vi "TLB Native Dynamic Events ver 0.15b.vi"() -> ()   [LabVIEW 2018]
uses:
  Labview Training Phase 2/Enum Controls/States for Action Engine.ctl
  TLB Type Definitions/State Type Definitions.ctl
  TLB Type Definitions/Intruction Type Definitions.ctl
  TLB Type Definitions/Encoder cluster.ctl
  TLB Type Definitions/PING CLUSTER.ctl
  <vilib>/Studica/Studica Toolkit/NavX/NavX.lvlib
  <vilib>/Studica/Studica Toolkit/Background/DIO Channel.ctl
  Underlying VI's/NavX VI/navX type def.ctl
  <vilib>/myRIO/Instrument Drivers/Utilities/Utilities.lvlib
  <vilib>/Studica/Studica Toolkit/Background/I2C Channel.ctl
  TLB Type Definitions/Vision cluster.ctl
  <vilib>/NI_Real-Time Target Support.lvlib
  TLB Type Definitions/Stepper cluster.ctl
  Experimental VI's/Archived VI's/MOTOR CONTROL NO PID Type Def.ctl
  Underlying VI's/I2C Master VI/I2C MASTER Type Def.ctl
  Underlying VI's/I2C Master VI/I2C_MASTER_WRITE_NEW Type Def.ctl
  <vilib>/userdefined/High Color/IMAQdx.ctl
  Underlying VI's/I2C Master VI/Arduino_Interfacing.ctl
  TLB Type Definitions/Yaw Cluster.ctl
  Experimental VI's/Archived VI's/MOTOR CONTROL NO PID AE DATA ENTRY MODE Type def.ctl
  Experimental VI's/Archived VI's/MOTOR CONTROL NO PID AE DIRECTIONS type def.ctl
  TLB Type Definitions/Time cluster.ctl
  TLB Type Definitions/Y Stepper cluster.ctl
  Underlying VI's/Modified webcam FGV/Webcam AE.ctl
  Underlying VI's/Elasped Timer/Elapsed timer control.ctl
  <vilib>/Utility/RT CPU Load.ctl
panel:
  out "Object Center Coordinates":cluster{"x":sgl, "y":sgl}
  out "Object detection cluster":T1
  out "Time up flag":bool
  out "Speed & distance":T2
  out "Task selection":u8
  in  "Object recognition mode":enum16{"Ball", "Soap", "Gel", "Pipe", "None"}(ring)
  out "NavX Readings":T3
  out "Arduino Data":T4
  out "CPU loads":T5[](array[typedef]) {"ISR (%)" format="%#.2f"; "Idle (%)" format="%#.2f"; "Background (%)" format="%#.2f"; "Normal (%)" format="%#.2f"; "Above Normal (%)" format="%#.2f"; "High (%)" format="%#.2g"; "Timed Structures (%)" format="%#.2g"; "Time Critical (%)" format="%#.2g"; "Total (%)" format="%#.2g"}
  out "TASK ENABLE":bool
  out "Rising Edge":bool
  in  "Green LED":bool
  out "Obstacle detected":bool
  out "I2C Error":errorcluster
  out "State Logic":T6=enum."Startup"
  out "elements":T7[](array[typedef])
  in  "STOP TASK":bool
  in  "OK Button":bool
  in  "STOP":bool
  out "error out":errorcluster
  out "Action Queue Items":i32
  out "State Logic Queue Items":i32
  out "Action Queues items":string[](array[string])=["Hardware reset", "Software reset", ""]
  out "Action State":string
  # "System Health Status Update"
  # "VISION"
  # "TLB FRAMEWORK STATUS"
  # "Test Programme written by Calvin Loke    Dated: 28 Aug 2019\nTest Programme revised by Dr Alex See   Dated 30 Aug 2019\n\nRevision date: 20/03/2020\nProgramme version:   TLB Native Dynamic Events ver 0.14a"
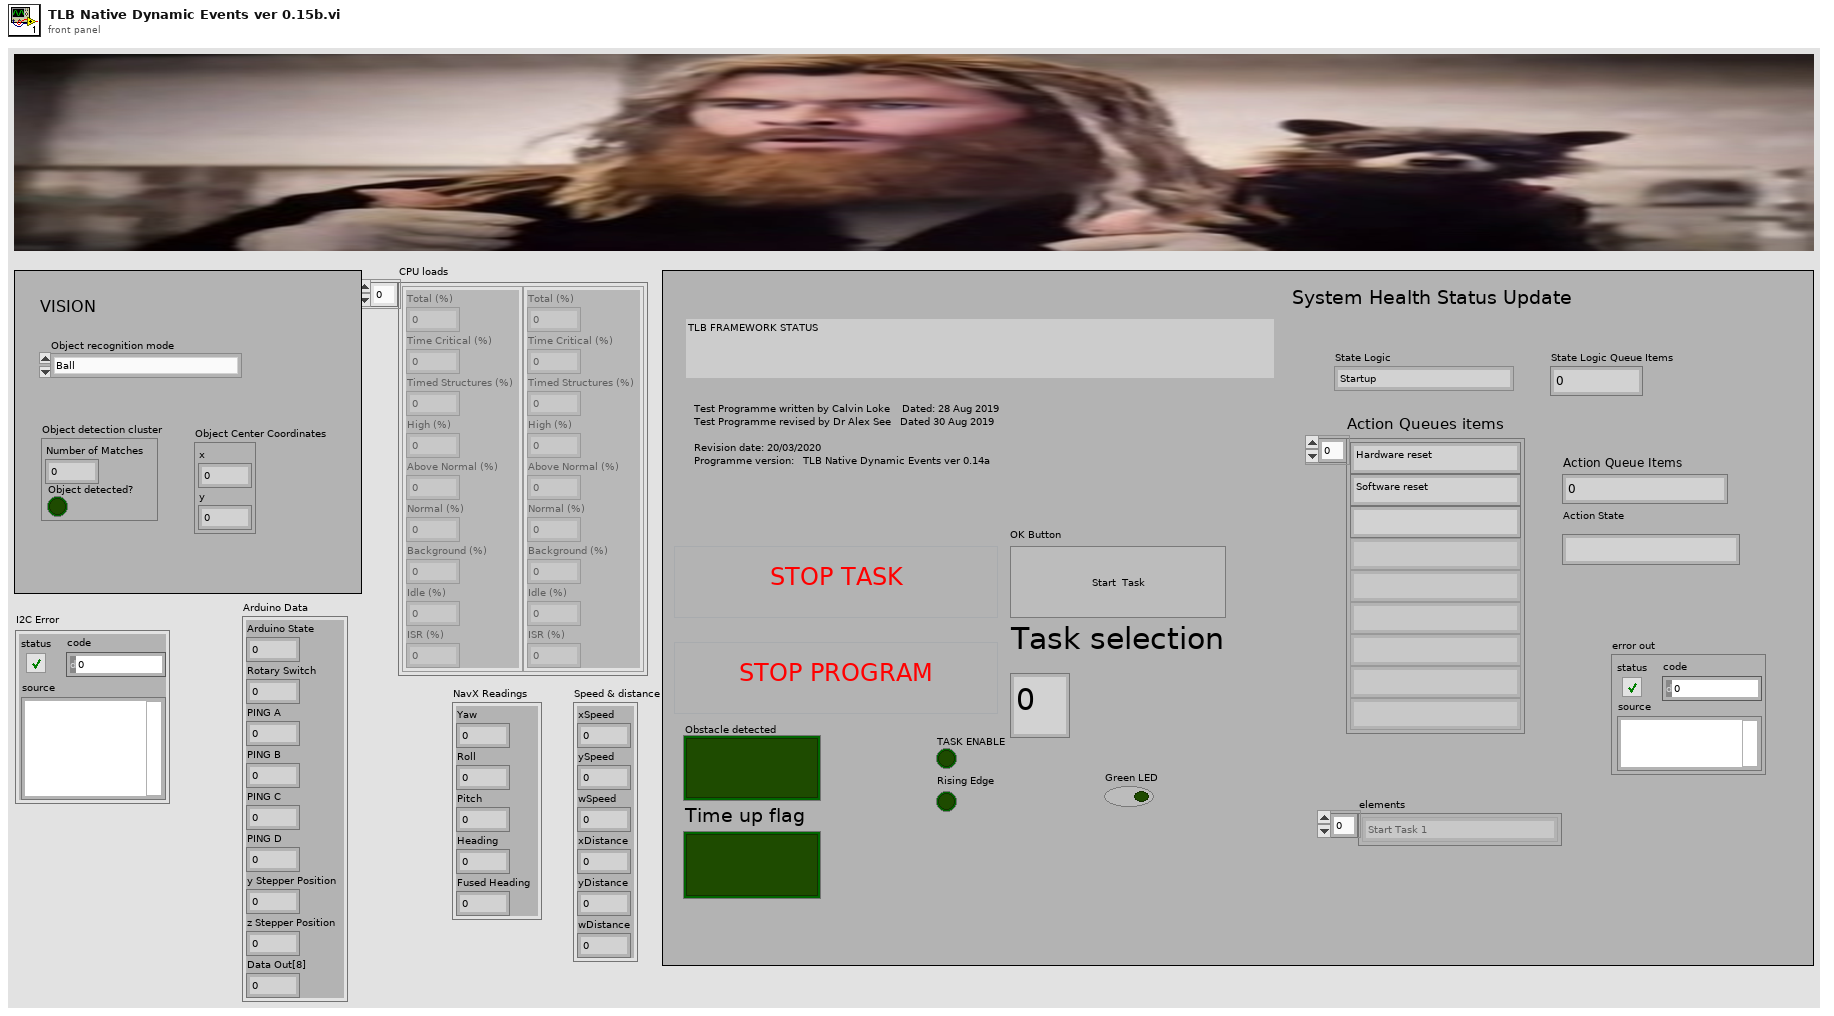
[diagram p1: front panel]
types:
  T1 = cluster{"Number of Matches":i32, "Object detected?":bool}
  T2 = cluster{"xSpeed":dbl, "ySpeed":dbl, "wSpeed":dbl, "xDistance":dbl, "yDistance":dbl, "wDistance":dbl}
  T3 = cluster{"Yaw":dbl, "Roll":dbl, "Pitch":dbl, "Heading":dbl, "Fused Heading":dbl}
  T4 = cluster{"Arduino State":u8, "Rotary Switch":u8, "PING A":u8, "PING B":u8, "PING C":u8, "PING D":u8, "y Stepper Position":u8, "z Stepper Position":u8, "Data Out[8]":u8}
  T5 = typedef "NI_Real-Time Target Support.lvlib/RT CPU Load.ctl" = cluster{"Total (%)":dbl, "Time Critical (%)":dbl, "Timed Structures (%)":dbl, "High (%)":dbl, "Above Normal (%)":dbl, "Normal (%)":dbl, "Background (%)":dbl, "Idle (%)":dbl, "ISR (%)":dbl}
  T6 = typedef "State Type Definitions.ctl" = enum16{"None", "Startup", "Move to Angle", "True Stop", "Idle", "Shutdown", "Task 1A", "Task 1B", "Task 2:Raise Arm", "Task 2:Sensor Mode", "Task 2:Reverse Mode", "Task 3", "Task 4_A", "Task 4_B", "Task 4_C", "Task 4_D", "Task 5A", "Task 5B", "Task 5C", "Task 5D", "Task 5E: POSITION ARM", "Task 5F: ARM GRAB HEIGHT", "Task 5G: CLOSE CLAW", "Task 5H: RAISE ARM", "Task 6_A", "Task 6_B", "Task 7", "Task 8A: RAISE ARM", "Task 8B: MOVE TO BOX", "Task 8C: CAM BURST", "Task 8D: PROCESS IMAGE", "Task 8E: ROBOT ADJUST", "Task 8F: CAM BURST 2", "Task 8G: PROCESS IMAGE 2", "Task 8H: ARM ADJUST", "Task 8I: ARM GRAB HEIGHT", "Task 8J: CLOSE CLAW", "Task 8K: RAISE MY SWORD", "Task 9A: Raise Arm", "Task 9B: Rotate to Angle", "Task 9C: Detect Box", "Task 9D: MOVE FORWARD", "Task 9E: MOVE LEFT", "Task 9F: SCAN IMAGE", "Task 9G: PROCESS COLOUR", "Task 9H: MOVE RIGHT", "Task 9I: SCAN IMAGE", "Task 9J: PROCESS COLOUR", "Task 9K: ROTATE 90 CW", "Task 9L: MOVE FORWARD", "Task 9M: MOVE RIGHT", "Task 9N: SCAN IMAGE", "Task 9O: PROCESS COLOUR", "Task 9P: MOVE RIGHT", "Task 9Q: SCAN IMAGE", "Task 9R: PROCESS COLOUR", "Task A1: Raise Arm", "Task A2: Rotate to Angle", "Task A3: Move Forward", "Task A4: Rotate CW 90"}
  T7 = typedef "Intruction Type Definitions.ctl" = enum16{"None", "Start Task 1", "Start Task 2", "Start Task 3", "Start Task 4", "Start Task 5", "Start Task 6", "Start Task 7", "Start Task 8 - BALL", "Start Task 8 - Gel", "Start Task 8 - Pipe", "Start Task 8 - Soap", "Start Task 9", "Start Task A", "Start Task B", "Exit"}
  T8 = typedef "Y Stepper cluster.ctl" = cluster{"yStepper desired":u8}
  T9 = typedef "Time cluster.ctl" = cluster{"Time up flag":bool, "SET TIME TO CHECK":dbl}
  T10 = typedef "Yaw Cluster.ctl" = cluster{"Yaw":dbl, "Compass":dbl}
  T11 = typedef "Stepper cluster.ctl" = cluster{"y Stepper Position":u8, "z Stepper Position":u8}
  T12 = typedef "DIO Channel.ctl" = enum16{"Not Connected", "A/DIO1", "A/DIO2", "A/DIO3", "A/DIO4", "A/DIO5", "A/DIO6", "A/DIO7", "A/DIO13", "B/DIO1", "B/DIO2", "B/DIO3", "B/DIO4", "B/DIO5", "B/DIO6", "B/DIO7", "B/DIO13", "C/DIO0", "C/DIO1", "C/DIO2", "C/DIO3", "C/DIO4", "C/DIO5", "C/DIO6", "C/DIO7"}
  T13 = typedef "Vision cluster.ctl" = cluster{"Recognized Object":bool, "Object X coordinate":dbl, "Object Y coordinate":dbl}
  T14 = typedef "PING CLUSTER.ctl" = cluster{"PING_A":u8, "PING_B":u8, "PING_C":u8, "PING_D":u8}
  T15 = typedef "Encoder cluster.ctl" = cluster{"xDistance":dbl, "yDistance":dbl, "wDistance":dbl}
  T16 = cluster{"DIO Channel":T12, "FPGA VI Reference Out":refnum<k20>}
  T17 = typedef "MOTOR CONTROL NO PID AE DATA ENTRY MODE Type def.ctl" = enum16{"Initialize", "Reset Encoders", "Write to motors", "Read from Encoders"}
  T18 = typedef "navX type def.ctl" = enum16{"Get i2C reference", "Read Values", "Zero Yaw"}
  T19 = typedef "Arduino_Interfacing.ctl" = enum16{"Initialize", "Write to Arduino", "Read From Arduino"}
  T20 = typedef "I2C Channel.ctl" = enum16{"Not Connected", "A", "B"}
  T21 = typedef "States for Action Engine.ctl" = enum16{"Initialize", "Write", "Read"}
  T22 = cluster{"I2C Ref Out":cluster{"I2C Channel":T20, "FPGA VI Reference Out":refnum<k20>}, "Connected":bool, "Slave Address (7-bit)":u8, "Registry":u8[]}
  T23 = typedef "IMAQ Image.ctl" = refnum<image>
  T24 = typedef "State Type Definitions.ctl" = enum16{"None", "Startup", "Move to Angle", "True Stop", "Idle", "Shutdown", "Task 1", "Task 2", "Task 3", "Task 4_A", "Task 4_B", "Task 4_C", "Task 4_D", "Task 5_A", "Task 5 _B", "Task 5_C", "Task 5_D", "Task 5_D_Error", "Task 5D_Error_Right", "Task 5D_Error_Left", "Task 5_E", "Task 5_F", "Task 5F_Error", "Task 5G", "Task 5H", "Task 5I", "Task 6_A", "Task 6_B", "Task 7", "Task 8", "Task 9", "Task A", "Task B"}
  T25 = typedef "MOTOR CONTROL NO PID AE DIRECTIONS type def.ctl" = enum16{"y-axis movement", "x-axis movement", "Rotate", "Stop"}
  T26 = typedef "Elapsed timer control.ctl" = enum16{"Start", "Pause", "Initialize"}
  T27 = typedef "I2C_MASTER_WRITE_NEW Type Def.ctl" = enum16{"Ultrasonic sensors", "Stepper origin", "zStepper 13.3k", "zStepper 13k", "zStepper 12k", "zStepper 11k", "zStepper 10k", "zStepper 9k", "zStepper 8k", "zStepper 7k", "zStepper 6k", "zStepper 5k", "zStepper 4k", "zStepper 3k", "zStepper 2k", "zStepper 1k", "zStepper 900", "zStepper 800", "zStepper 700", "zStepper 600", "zStepper 500", "zStepper 400", "zStepper 300", "zStepper 200", "zStepper 100", "zStepper 0", "yStepper control", "Open Claw", "Close Claw", "Soft Reset"}
  T28 = typedef "Webcam AE.ctl" = enum16{"Initialize Camera", "Open Camera", "Continuous Acquisition", "Close Camera", "Retrieve Image", "Dispose Camera Image Buffer"}
  T29 = typedef "IMAQdx.ctl" = refnum<k21>
  T30 = typedef "Webcam AE.ctl" = enum16{"Initialize Camera", "Open Camera", "Continuous Acquisition", "Close Camera", "Retrieve Image", "Dispose Image Buffers"}
  T31 = typedef "MOTOR CONTROL NO PID Type Def.ctl" = enum16{"Init", "Front Back", "Left Right", "Rotate", "Stop", "Latch"}
  T32 = typedef "I2C MASTER Type Def.ctl" = enum16{"Last State", "Mode 0", "Mode 1", "Mode 2", "Mode 3", "Mode 4", "Mode 5", "Mode 6", "Mode 7", "Mode 8", "Mode 9", "Mode 10"}
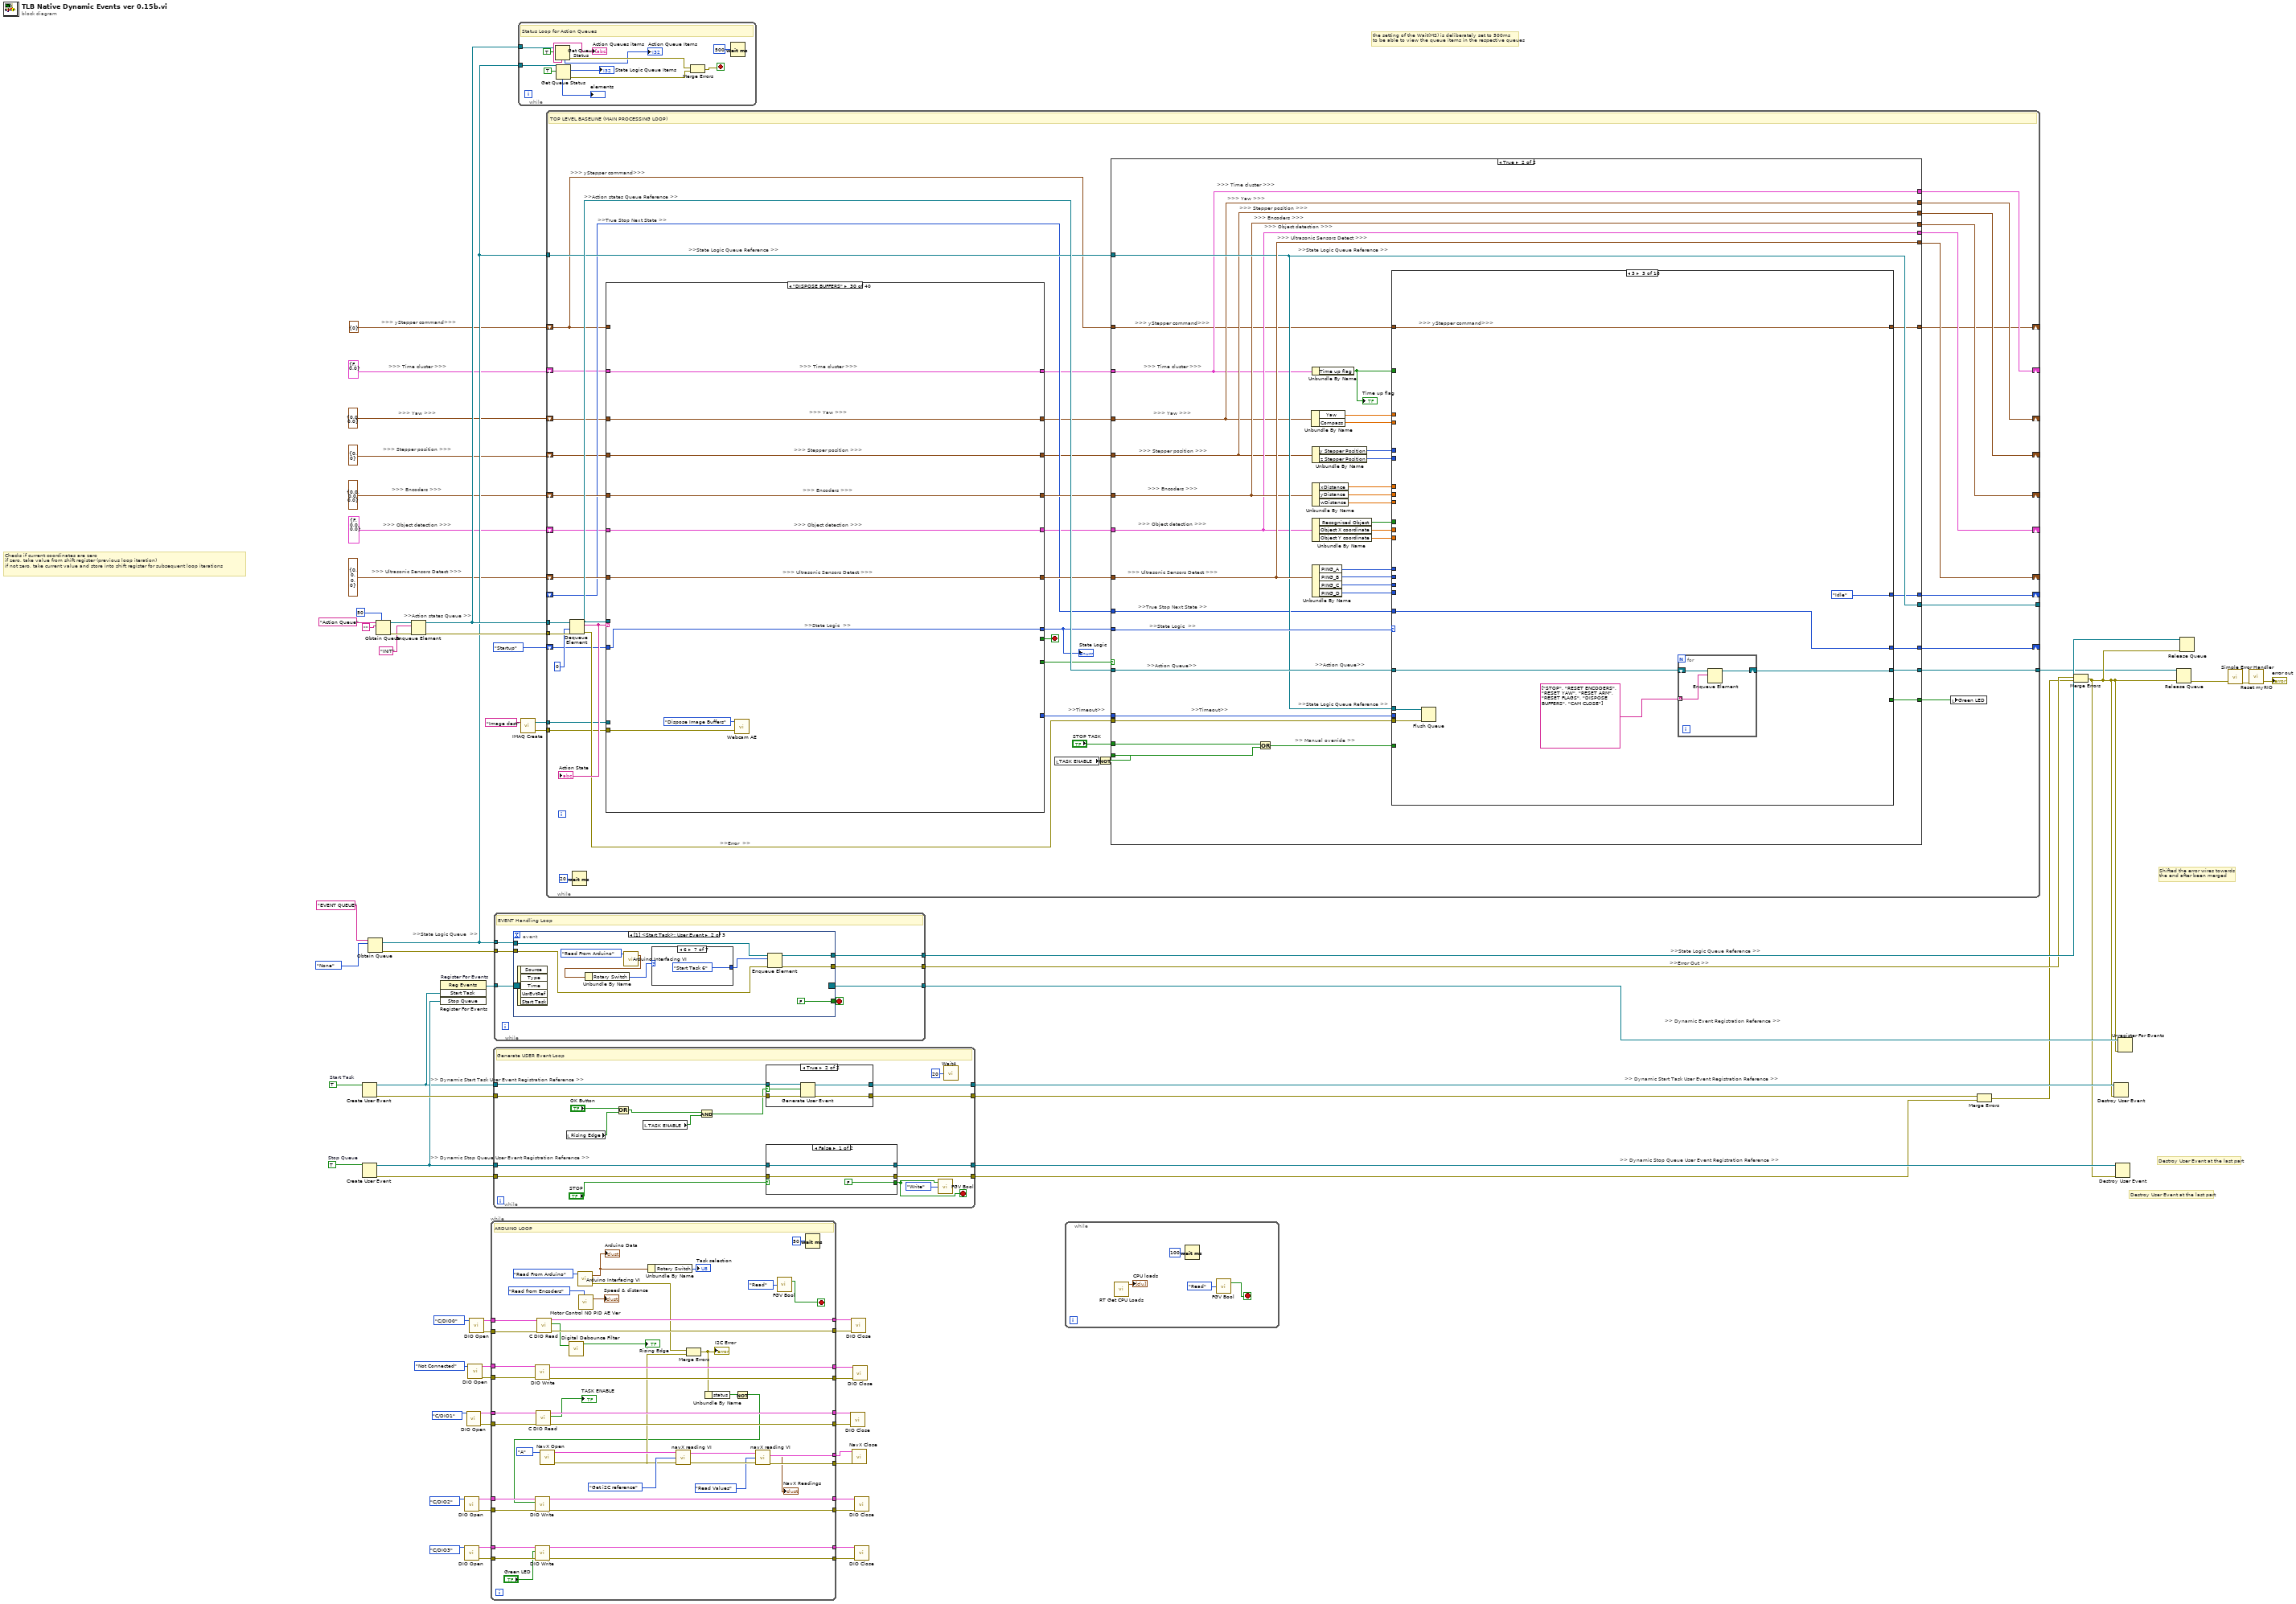
[diagram p0: block diagram]
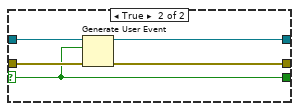
[diagram p2: hidden frame]
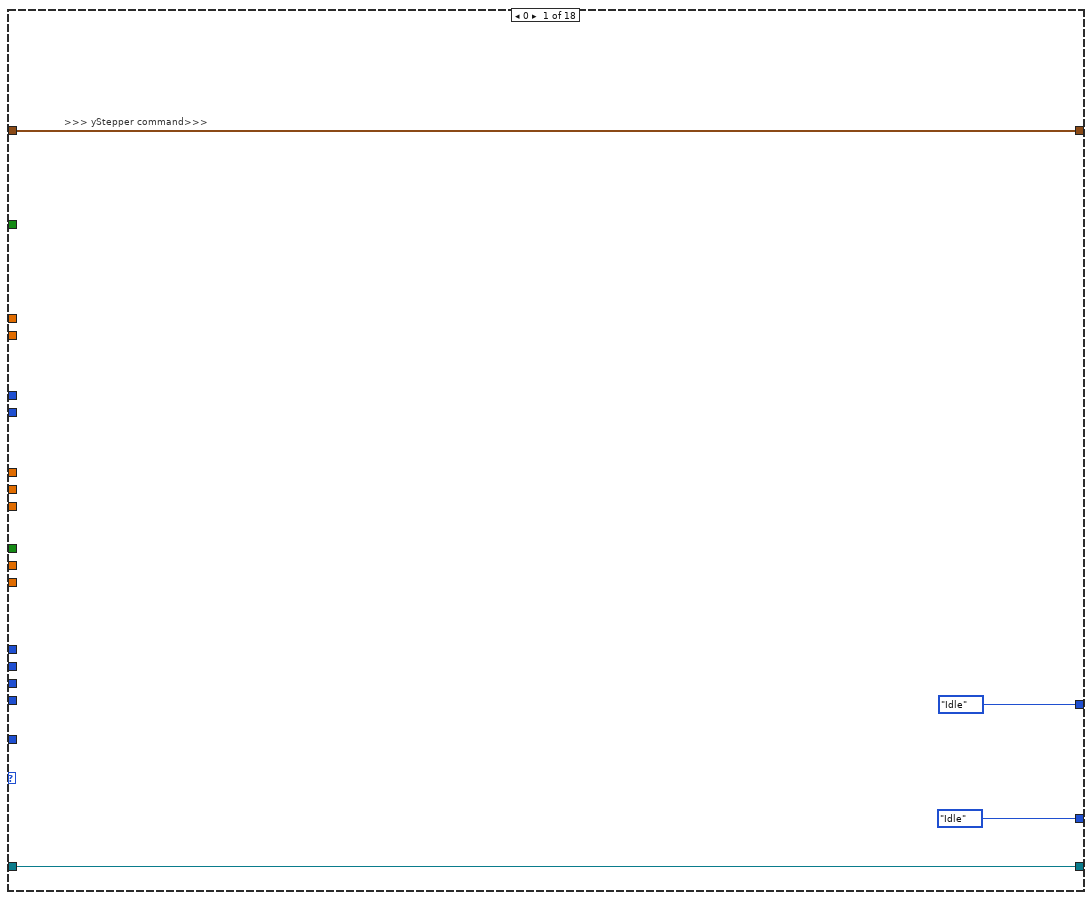
[diagram p5: hidden frame]
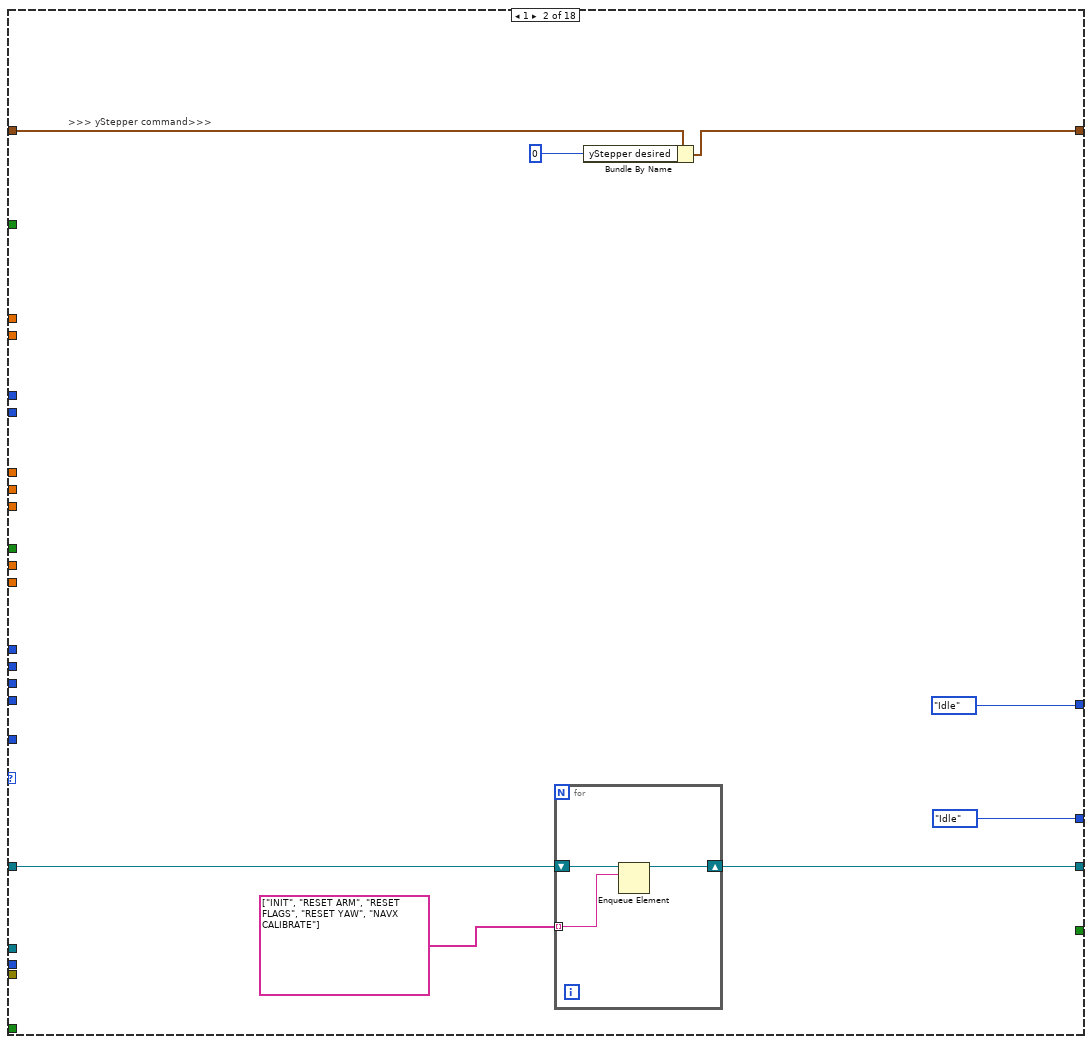
[diagram p6: hidden frame]
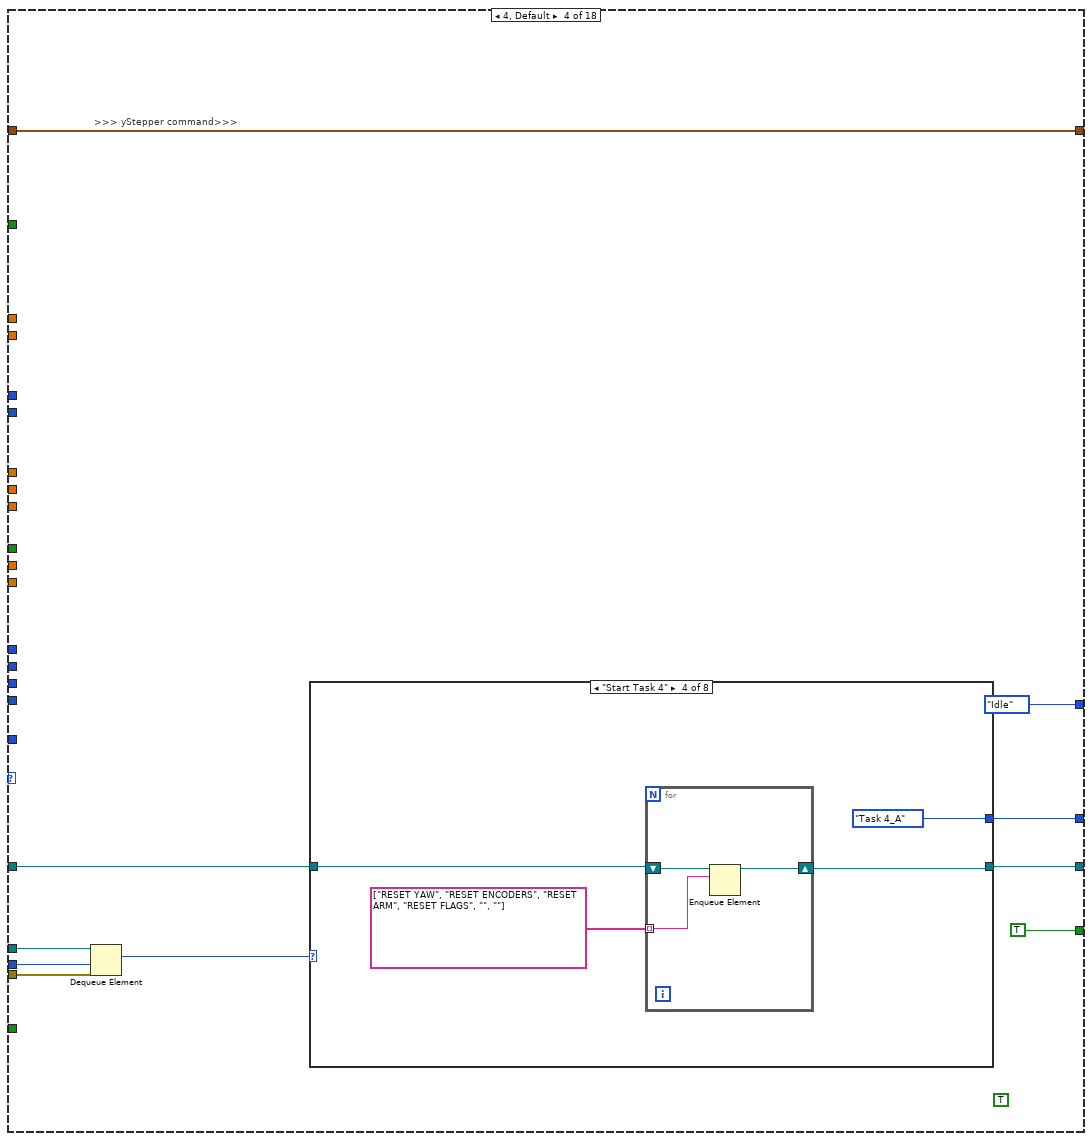
[diagram p7: hidden frame]
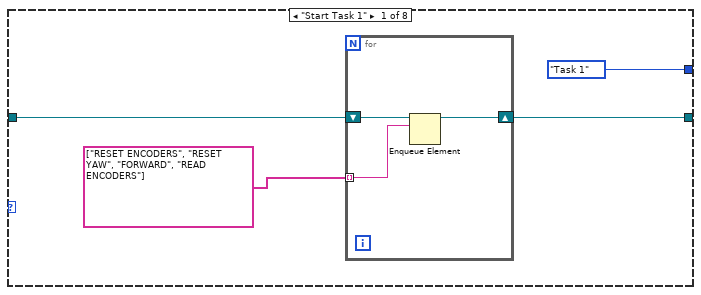
[diagram p8: hidden frame]
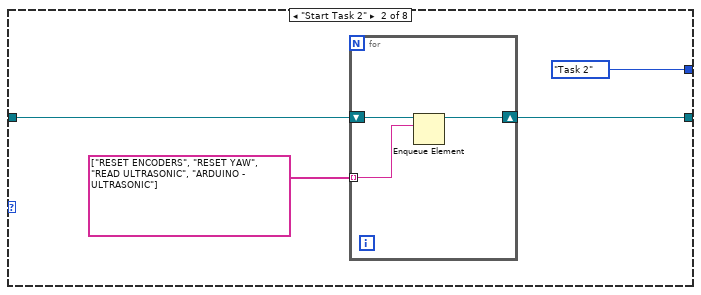
[diagram p9: hidden frame]
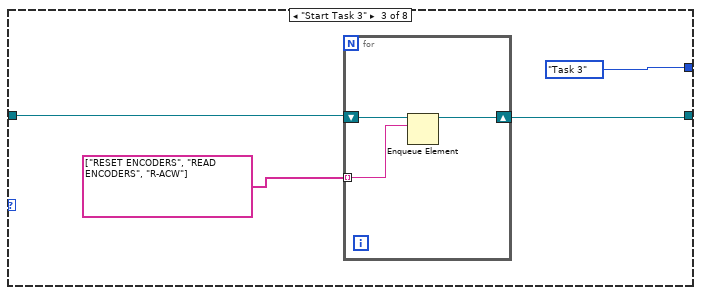
[diagram p10: hidden frame]
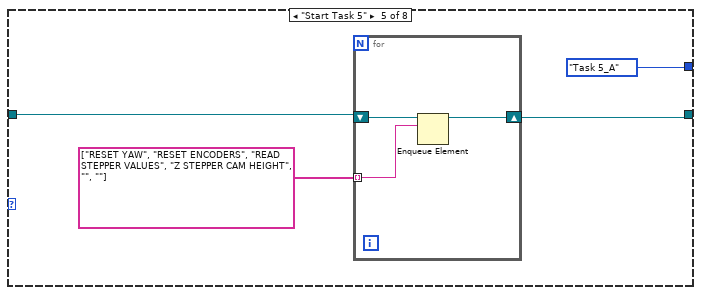
[diagram p11: hidden frame]
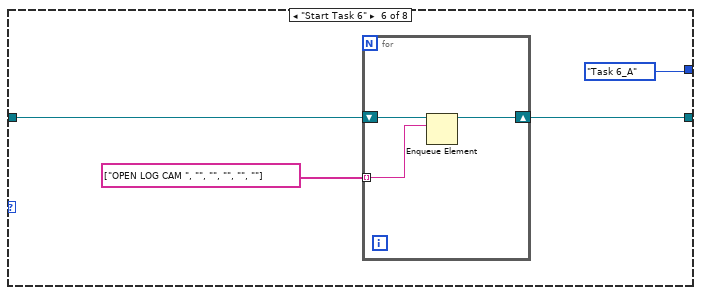
[diagram p12: hidden frame]
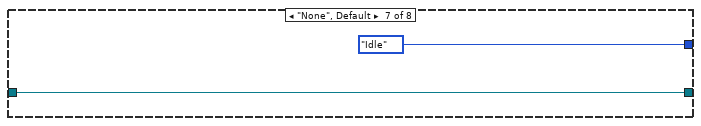
[diagram p13: hidden frame]
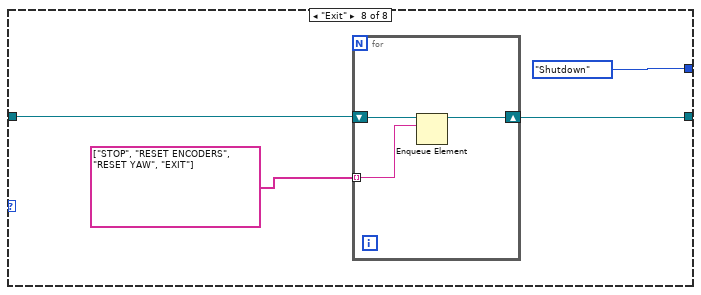
[diagram p14: hidden frame]
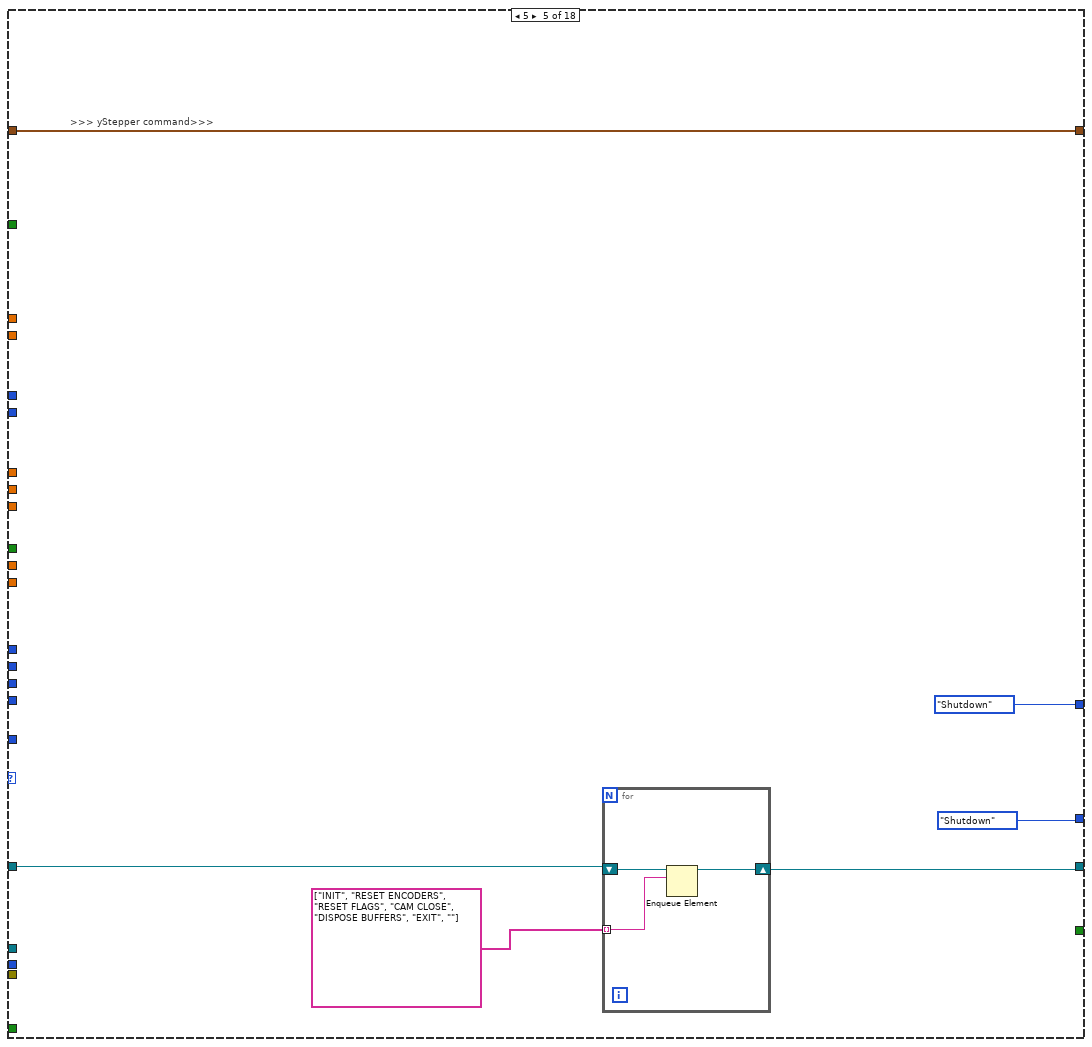
[diagram p15: hidden frame]
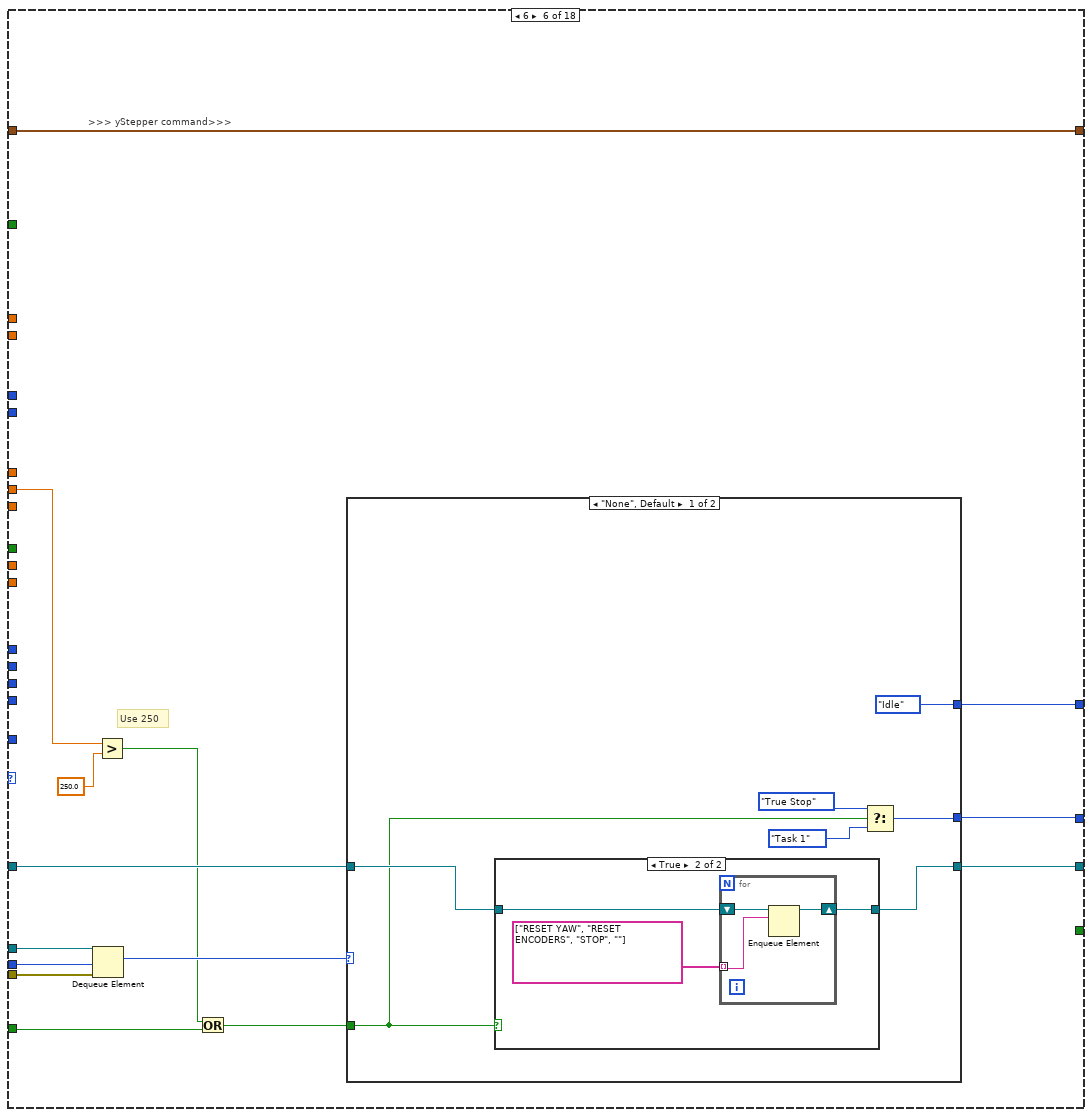
[diagram p16: hidden frame]
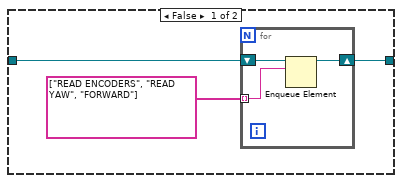
[diagram p17: hidden frame]
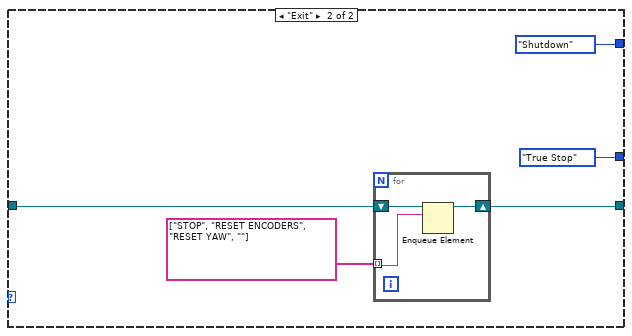
[diagram p18: hidden frame]
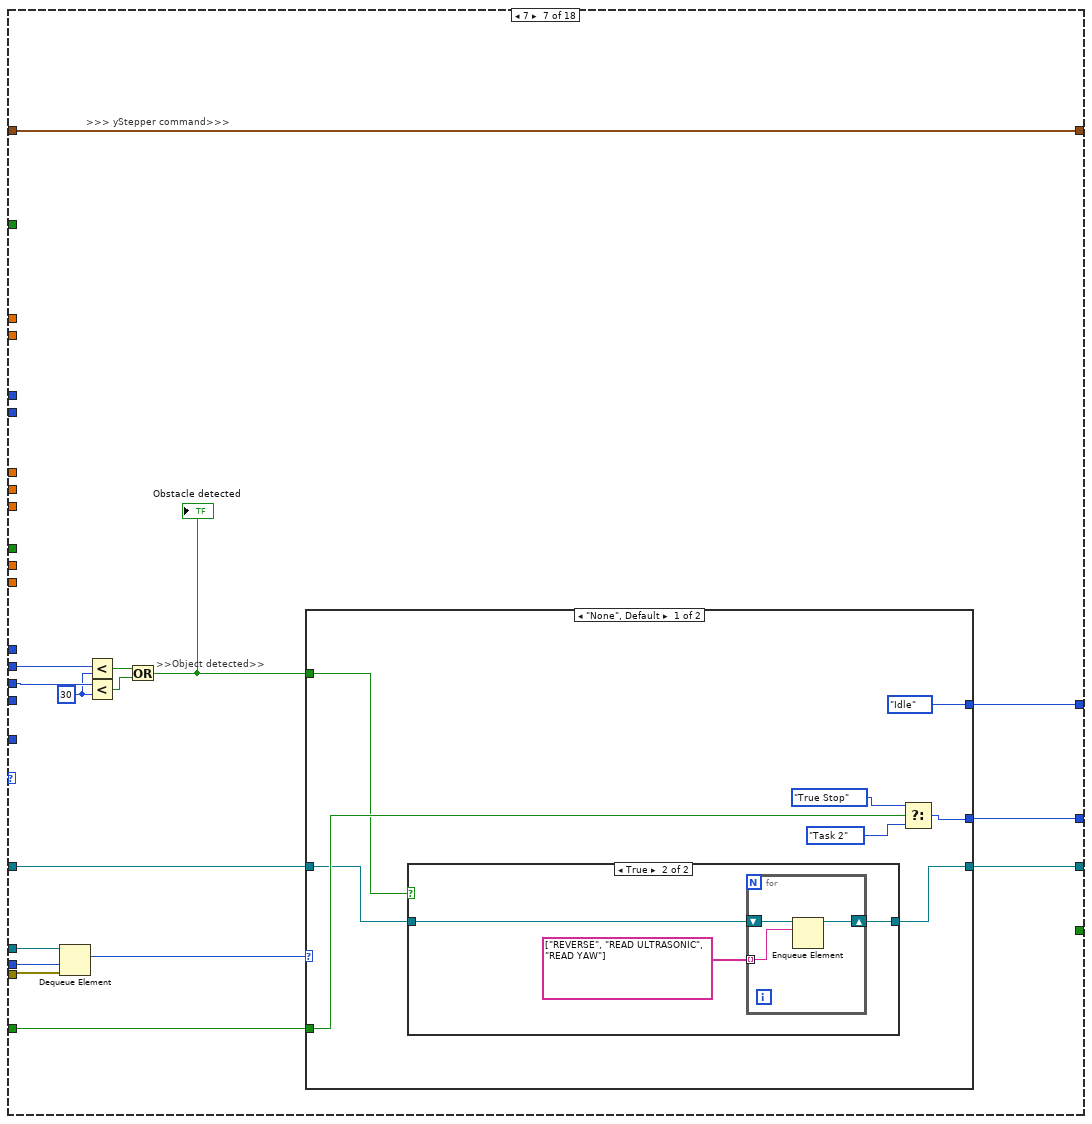
[diagram p19: hidden frame]
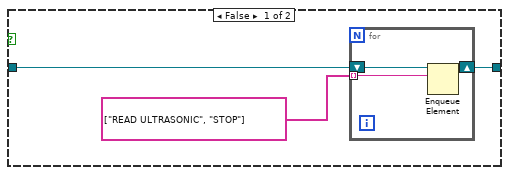
[diagram p20: hidden frame]
diagram:
  w70 = TRUE  # Stop Queue
  w69 = TRUE  # Start Task
  # "Checks if current coordinates are zero\nif zero, take value from shift register (previous loop iteration)\nif not zero, take current value and store into shift register for subsequent loop iterations"
  # ">>> yStepper command>>>"
  # ">>> Time cluster >>>"
  # ">>> Yaw >>>"
  # ">>> Stepper position >>>"
  # ">>> Encoders >>>"
  # ">>> Object detection >>>"
  # ">>> Ultrasonic Sensors Detect >>>"
  # "the setting of the Wait(MS) is deliberately set to 500ms\nto be able to view the queue items in the respective queues"
  # ">>Error Out >>"
  # ">> Dynamic Stop Queue User Event Registration Reference >>"
  # ">> Dynamic Start Task User Event Registration Reference >>"
  # ">> Dynamic Stop Queue User Event Registration Reference >>"
  # ">> Dynamic Start Task User Event Registration Reference >>"
  # ">> Dynamic Event Registration Reference >>"
  # ">>Action states Queue >>"
  # ">>State Logic Queue  >>"
  # ">>State Logic Queue Reference >>"
  # "Destroy User Event at the last part"
  # "Destroy User Event at the last part"
  # "Shifted the error wires towards\nthe end after been merged"
  n1 = Create User Event(user event datatype=w69) -> (user event=w61:refnum<user-event>, error out=w66:errorcluster)  [unwired: 1 in]
  n2 = Create User Event(user event datatype=w70) -> (user event=w62:refnum<user-event>, error out=w65:errorcluster)  [unwired: 1 in]
  n3 = Obtain Queue(name (unnamed)="EVENT QUEUE", element data type=Intruction_Type_Definitions."None" ("Enum")) -> (queue out=w47:refnum<queue>, error out=w53:errorcluster)  [unwired: 3 in, 1 out]
  n4 = Obtain Queue(max queue size (-1, unlimited)=50, name (unnamed)="Action Queue", element data type="") -> (queue out=w56:refnum<queue>, error out=w52:errorcluster)  [unwired: 2 in, 1 out]
  n5 = Enqueue Element(queue=w56, element="INIT", error in (no error)=w52) -> (queue out=w48:refnum<queue>, error out=w51:errorcluster)  [unwired: 1 in, 1 out]
  n6 = register-events "Register For Events"(w61, w62) -> (reference out=w60:refnum<event-registration>)  [unwired: 2 in, 1 out]
  n7 = call <vilib>:"DIO Open.vi"("DIO Channel"=DIO_Channel."C/DIO2") -> ("error out"=w14:errorcluster, "DIO Info Out"=w15:T16)  [unwired: 9 in]
  n8 = call <vilib>:"DIO Open.vi"("DIO Channel"=DIO_Channel."C/DIO3") -> ("error out"=w9:errorcluster, "DIO Info Out"=w10:T16)  [unwired: 9 in]
  n9 = call <vilib>:"DIO Open.vi"("DIO Channel"=DIO_Channel."C/DIO1") -> ("error out"=w25:errorcluster, "DIO Info Out"=w26:T16)  [unwired: 9 in]
  n10 = call <vilib>:"DIO Open.vi"("DIO Channel"=DIO_Channel."Not Connected") -> ("error out"=w30:errorcluster, "DIO Info Out"=w32:T16)  [unwired: 9 in]
  n11 = call <vilib>:"DIO Open.vi"("DIO Channel"=DIO_Channel."C/DIO0") -> ("error out"=w35:errorcluster, "DIO Info Out"=w38:T16)  [unwired: 9 in]
  n12 = while {
    tunnel: w38 -> [w113]
    tunnel: [w112] -> w36
    tunnel: w35 -> [w111]
    tunnel: [w110] -> w34
    tunnel: w32 -> [w107]
    tunnel: [w106] -> w31
    tunnel: w30 -> [w105]
    tunnel: [w104] -> w29
    tunnel: [w103] -> w27
    tunnel: w26 -> [w102]
    tunnel: w25 -> [w101]
    tunnel: [w100] -> w24
    tunnel: w15 -> [w94]
    tunnel: w14 -> [w93]
    tunnel: [w92] -> w13
    tunnel: [w91] -> w12
    tunnel: w10 -> [w90]
    tunnel: w9 -> [w89]
    tunnel: [w88] -> w8
    tunnel: [w87] -> w7
    tunnel: [w81] -> w4
    tunnel: [w80] -> w5
    stop <- w115 stop-if-true
    # "ARDUINO LOOP"
    n13 = call <vilib>:"DIO Write.vi"("error in (no error)"=w89, "Input"="Green LED", "DIO Info In"=w90) -> ("error out"=w87:errorcluster, "DIO Info Out"=w88:T16)  [unwired: 7 in]
    n14 = call <vilib>:"DIO Write.vi"("error in (no error)"=w105, "DIO Info In"=w107) -> ("error out"=w104:errorcluster, "DIO Info Out"=w106:T16)  [unwired: 8 in]
    n15 = call <vilib>:"C DIO Read.vi"("error in (no error)"=w101, "DIO Info In in"=w102) -> ("error out"=w100:errorcluster, "IN"=→"TASK ENABLE":bool, "DIO Info In out"=w103:T16)  [unwired: 7 in]
    n16 = call <vilib>:"C DIO Read.vi"("error in (no error)"=w111, "DIO Info In in"=w113) -> ("error out"=w110:errorcluster, "IN"=w109:bool, "DIO Info In out"=w112:T16)  [unwired: 7 in]
    n17 = call <vilib>:"NavX Open.vi"("I2C Channel"=I2C_Channel."A") -> ("error out"=w96:errorcluster, "NavX Info"=w98:T22)  [unwired: 9 in]
    n18 = call "Digital Debounce Filter.vi"("Boolean input"=w109) -> ("Rising Edge"=→"Rising Edge":bool)  [unwired: 1 in, 2 out]
    n19 = call "Arduino Interfacing VI.vi"("AE Mode"=Arduino_Interfacing."Read From Arduino") -> ("error out"=w84:errorcluster, "Arduino Data"=w77:T4)  [unwired: 3 in]
    "Arduino Data" <- w77
    n20 = call "Motor Control NO PID AE Ver.vi"("AE Mode"=MOTOR_CONTROL_NO_PID_AE_DATA_ENTRY_MODE_Type_def."Read from Encoders") -> ("Speed & distance"=→"Speed & distance":T2)  [unwired: 4 in, 1 out]
    n21 = Unbundle By Name(w77) -> ("Rotary Switch"=→"Task selection":u8)
    n22 = call "navX reading VI.vi"("NavX Info In"=w98, "Mode"=navX_type_def."Get i2C reference", "error in (no error)"=w96) -> ("NavX Info Out"=w83:T22, "Error Out"=w82:errorcluster)  [unwired: 2 out]
    n23 = Merge Errors(w84, w96) -> (w73:errorcluster)
    "I2C Error" <- w73
    n24 = Unbundle By Name(w73) -> ("status"=w72:bool)
    n25 = Not(x=w72) -> (.not. x?=w71:bool)
    n26 = call <vilib>:"DIO Write.vi"("error in (no error)"=w93, "Input"=w71, "DIO Info In"=w94) -> ("error out"=w91:errorcluster, "DIO Info Out"=w92:T16)  [unwired: 7 in]
    n27 = call "navX reading VI.vi"("NavX Info In"=w83, "Mode"=navX_type_def."Read Values", "error in (no error)"=w82) -> ("NavX Info Out"=w81:T22, "NavX Readings"=→"NavX Readings":T3, "Error Out"=w80:errorcluster)  [unwired: 1 out]
    n28 = call "FGV Bool.vi"("Init/Read/Write State"=States_for_Action_Engine."Read") -> ("Output node"=w115:bool)  [unwired: 2 in, 1 out]
    n29 = Wait (ms)(milliseconds to wait=u32 50) -> ()  [unwired: 1 out]
  }
  n30 = while {
    tunnel: w61 -> [w133]
    tunnel: w62 -> [w132]
    tunnel: [w131] -> w68
    tunnel: [w130] -> w67
    tunnel: w66 -> [w129]
    tunnel: [w128] -> w64
    tunnel: w65 -> [w127]
    tunnel: [w126] -> w63
    stop <- w124 stop-if-true
    # "Generate USER Event Loop"
    n31 = local read "Rising Edge"() -> (w120:bool)
    n32 = Or(x="OK Button", y=w120) -> (x .or. y?=w119:bool)
    n33 = local read "TASK ENABLE"() -> (w118:bool)
    n34 = And(x=w119, y=w118) -> (x .and. y?=w117:bool)
    n35 = case shown="True" w117 {
      selector: w117 -> [_ w144]
      tunnel: w133 -> [w143 w148]
      tunnel: [w143 w147] -> w130
      tunnel: w129 -> [w142 w146]
      tunnel: [w142 w145] -> w128
      frame False {
      }
      frame True {
        n36 = Generate User Event(user event=w148, event data cluster=w144, error in=w146) -> (user event out=w147:refnum<user-event>, error out=w145:errorcluster)  [unwired: 1 in]
      }
    }
    n37 = case shown="False" "STOP" {
      selector: "STOP" -> [_ w137]
      tunnel: w132 -> [w136 w141]
      tunnel: [w136 w140] -> w131
      tunnel: w127 -> [w135 w139]
      tunnel: [w135 w138] -> w126
      tunnel: [FALSE w137] -> w124
      frame False {
      }
      frame True {
        n38 = Generate User Event(user event=w141, event data cluster=w137, error in=w139) -> (user event out=w140:refnum<user-event>, error out=w138:errorcluster)  [unwired: 1 in]
      }
    }
    n39 = call "FGV Bool.vi"("Init/Read/Write State"=States_for_Action_Engine."Write", "Input Node"=w124) -> ()  [unwired: 1 in, 2 out]
    n40 = call "Wait4"("Count(uSec)"=u32 20) -> ()  [unwired: 1 out]
  }
  n41 = while {
    tunnel: w60 -> [w155]
    tunnel: [w154] -> w59
    tunnel: w47 -> [w152]
    tunnel: [w151] -> w58
    tunnel: w53 -> [w150]
    tunnel: [w149] -> w50
    stop <- w153 stop-if-true
    # "EVENT Handling Loop"
    n42 = event shown="[1] <Start Task>: User Event" {
      selector: w155 -> [_ _ _]
      dyn-events: [_ _ _] -> w154
      timeout: _ -> [_ _ _]
      tunnel: [FALSE FALSE w183] -> w153
      tunnel: w152 -> [w160 w169 w181]
      tunnel: [w159 w168 w182] -> w151
      tunnel: w150 -> [w158 w167 w180]
      tunnel: [w157 w166 w179] -> w149
      event Timeout {
        n43 = event-data() -> ()  [unwired: 1 in, 3 out]
        n44 = Enqueue Element(queue=w160, element=Intruction_Type_Definitions."None" ("Enum"), error in (no error)=w158) -> (queue out=w159:refnum<queue>, error out=w157:errorcluster)  [unwired: 1 in, 1 out]
      }
      event User Event {
        n45 = event-data() -> ()  [unwired: 1 in, 5 out]
        n46 = call "Arduino Interfacing VI.vi"("AE Mode"=Arduino_Interfacing."Read From Arduino") -> ("Arduino Data"=w163:T4)  [unwired: 3 in, 1 out]
        n47 = Unbundle By Name(w163) -> ("Rotary Switch"=w162:u8)
        n48 = case shown="6" w162 {
          tunnel: [Intruction_Type_Definitions."None" ("Enum") Intruction_Type_Definitions."Start Task 1" ("Enum") Intruction_Type_Definitions."Start Task 2" ("Enum") Intruction_Type_Definitions."Start Task 3" ("Enum") Intruction_Type_Definitions."Start Task 4" ("Enum") Intruction_Type_Definitions."Start Task 5" ("Enum") Intruction_Type_Definitions."Start Task 6" ("Enum")] -> w165
          frame 0, Default {
          }
          frame 1 {
          }
          frame 2 {
          }
          frame 3 {
          }
          frame 4 {
          }
          frame 5 {
          }
          frame 6 {
          }
        }
        n49 = Enqueue Element(queue=w169, element=w165, error in (no error)=w167) -> (queue out=w168:refnum<queue>, error out=w166:errorcluster)  [unwired: 1 in, 1 out]
      }
      event User Event {
        n50 = event-data() -> ("Stop Queue"=w183:bool)  [unwired: 1 in, 4 out]
        n51 = Enqueue Element At Opposite End(queue=w181, element=Intruction_Type_Definitions."Exit" ("Enum"), error in (no error)=w180) -> (queue out=w182:refnum<queue>, error out=w179:errorcluster)  [unwired: 1 in, 1 out]
      }
    }
  }
  n52 = while {
    tunnel: w48 -> [w193]
    tunnel: w47 -> [w190]
    stop <- w187 stop-if-true
    # "Status Loop for Action Queues"
    n53 = Get Queue Status(queue=w193, return elements? (F)=TRUE) -> (error out=w189:errorcluster, # elements in queue=→"Action Queue Items":i32, elements=→"Action Queues items":string[])  [unwired: 1 in, 5 out]
    n54 = Get Queue Status(queue=w190, return elements? (F)=TRUE) -> (# pending remove=→"State Logic Queue Items":i32, error out=w188:errorcluster, elements=→"elements":T7[])  [unwired: 1 in, 5 out]
    n55 = Merge Errors(w189, w188) -> (w187:errorcluster)
    n56 = Wait (ms)(milliseconds to wait=u32 500) -> ()  [unwired: 1 out]
  }
  n57 = call "IMAQ Create"("Image Name"="Image dest") -> ("New Image"=w19:T23, "error out"=w18:errorcluster)  [unwired: 4 in]
  n58 = while {
    tunnel: w47 -> [w227]
    tunnel: w48 -> [w239]
    tunnel: w51 -> [w237]
    tunnel: [w236] -> _
    tunnel: [w235] -> w41
    shift-right: [w228] -> _
    shift-left: T14 {"PING_A"=0, "PING_B"=0, "PING_C"=0, "PING_D"=0} -> [w230]
    shift-right: [w221] -> _
    shift-left: State_Type_Definitions."Startup" ("Enum") -> [w224]
    shift-right: [w217] -> _
    shift-left: T15 {"xDistance"=0.0, "yDistance"=0.0, "wDistance"=0.0} -> [w219]
    shift-right: [w214] -> _
    shift-left: _ -> [w213]
    tunnel: w19 -> [w212]
    tunnel: w18 -> [w211]
    shift-right: [w208] -> _
    shift-left: T13 {"Recognized Object"=FALSE, "Object X coordinate"=0.0, "Object Y coordinate"=0.0} -> [w210]
    shift-right: [w205] -> _
    shift-left: T11 {"y Stepper Position"=0, "z Stepper Position"=0} -> [w207]
    shift-right: [w202] -> _
    shift-left: T10 {"Yaw"=0.0, "Compass"=0.0} -> [w204]
    shift-right: [w199] -> _
    shift-left: T9 {"Time up flag"=FALSE, "SET TIME TO CHECK"=0.0} -> [w201]
    shift-right: [w197] -> _
    shift-left: T8 {"yStepper desired"=0} -> [w198]
    stop <- w226 stop-if-true
    # ">>> yStepper command>>>"
    # ">>True Stop Next State >>"
    # ">>Error  >>"
    # ">>Timeout>>"
    # ">>Action states Queue Reference >>"
    # ">>State Logic Queue Reference >>"
    # "TOP LEVEL BASELINE (MAIN PROCESSING LOOP)"
    n59 = Dequeue Element(queue=w239, timeout in ms (-1)=0, error in (no error)=w237) -> (queue out=w231:refnum<queue>, element=w238:string, error out=w232:errorcluster)  [unwired: 1 out]
    "Action State" <- w238
    n60 = Wait (ms)(milliseconds to wait=u32 20) -> ()  [unwired: 1 out]
    n61 = case shown="\"DISPOSE BUFFERS\"" w238 {
      tunnel: [_ _ _ _ _ _ _ _ _ _ _ _ _ _ _ _ 0 w1147 _ _ _ _ _ _ _ _ _ _ _ _ _ _ _ _ _ _ _ _ _ _] -> w234
      tunnel: w231 -> [_ _ _ _ _ _ _ _ _ _ _ _ _ _ _ _ _ _ _ _ _ _ _ _ _ _ _ _ _ _ _ _ _ _ _ _ _ _ _ _]
      tunnel: w230 -> [w962 w970 w981 w992 w1002 w1012 w1023 w1034 w1044 w1050 w1064 w1077 w1088 w1096 w1120 w1129 w1139 w1148 w1156 w1164 w1193 w1203 w1210 w1218 w1230 w1242 w1251 w1259 w1275 w1283 w1293 w1302 w1311 w1320 w1326 w1337 w1352 w1357 w1368 w1378]
      tunnel: [w962 w970 w981 w992 w1002 w1012 w1023 w1034 w1044 w1050 w1064 w1078 w1088 w1096 w1121 w1129 w1139 w1148 w1156 w1164 w1192 w1203 w1210 w1218 w1230 w1242 w1251 w1259 w1275 w1283 w1293 w1302 w1311 w1320 w1326 w1337 w1352 w1357 w1368 w1378] -> w229
      tunnel: [TRUE TRUE _ _ _ _ _ _ _ _ _ _ _ _ _ _ _ _ _ _ _ _ _ _ _ _ _ _ _ _ _ _ _ _ _ _ _ _ _ _] -> w226
      tunnel: w224 -> [w960 w968 w980 w991 w1001 w1011 w1022 w1033 w1043 w1049 w1063 w1076 w1087 w1095 w1119 w1128 w1136 w1145 w1155 w1163 w1191 w1202 w1209 w1217 w1229 w1241 w1250 w1258 w1274 w1282 w1292 w1301 w1310 w1319 w1325 w1336 w1351 w1356 w1367 w1377]
      tunnel: [_ _ _ _ _ _ _ _ _ _ _ _ _ _ _ _ _ TRUE _ _ _ _ _ _ _ _ _ _ _ _ _ _ _ _ _ _ _ _ _ _] -> w223
      tunnel: [w960 w968 w980 w991 w1001 w1011 w1022 w1033 w1043 w1049 w1063 w1076 w1087 w1095 w1119 w1128 w1136 w1145 w1155 w1163 w1191 w1202 w1209 w1217 w1229 w1241 w1250 w1258 w1274 w1282 w1292 w1301 w1310 w1319 w1325 w1336 w1351 w1356 w1367 w1377] -> w222
      tunnel: w219 -> [w959 w967 w979 w990 w1000 w1010 w1021 w1032 w1042 w1051 w1062 w1075 w1089 w1097 w1118 w1130 w1135 w1144 w1157 w1165 w1181 w1201 w1212 w1219 w1231 w1243 w1252 w1260 w1276 w1285 w1295 w1304 w1313 w1322 w1328 w1339 w1354 w1359 w1370 w1380]
      tunnel: [w959 w967 w979 w990 w1000 w1010 w1021 w1032 w1042 w1051 w1061 w1075 w1089 w1097 w1117 w1130 w1135 w1144 w1157 w1165 w1180 w1201 w1212 w1219 w1231 w1243 w1252 w1260 w1276 w1285 w1295 w1304 w1313 w1322 w1328 w1339 w1354 w1359 w1370 w1380] -> w218
      tunnel: w212 -> [w954 _ _ _ _ _ _ _ _ _ _ _ _ _ _ _ _ _ _ _ _ _ _ _ _ _ _ _ w1270 _ _ _ _ _ _ _ _ _ _ _]
      tunnel: w211 -> [_ _ _ _ _ _ _ _ _ _ _ _ _ _ _ _ _ _ _ _ _ _ _ _ _ _ w1244 _ w1272 w1281 _ _ _ _ _ _ _ _ _ _]
      tunnel: w210 -> [w958 w966 w978 w989 w999 w1009 w1020 w1031 w1040 w1048 w1060 w1074 w1082 w1094 w1109 w1127 w1134 w1143 w1154 w1162 w1186 w1199 w1211 w1216 w1228 w1240 w1246 w1257 w1267 w1284 w1294 w1303 w1312 w1321 w1327 w1338 w1353 w1358 w1369 w1379]
      tunnel: [w958 w966 w978 w989 w999 w1009 w1020 w1031 w1040 w1048 w1060 w1074 w1082 w1094 w1108 w1127 w1134 w1143 w1154 w1162 w1185 w1199 w1211 w1216 w1228 w1240 w1246 w1257 w1266 w1284 w1294 w1303 w1312 w1321 w1327 w1338 w1353 w1358 w1369 w1379] -> w209
      tunnel: w207 -> [w957 w965 w977 w988 w998 w1008 w1019 w1030 w1039 w1047 w1059 w1073 w1090 w1093 w1114 w1126 w1133 w1142 w1153 w1161 w1176 w1198 w1208 w1215 w1227 w1239 w1249 w1256 w1277 w1286 w1291 w1300 w1309 w1318 w1329 w1340 w1350 w1360 w1371 w1381]
      tunnel: [w957 w965 w977 w988 w998 w1008 w1019 w1030 w1039 w1047 w1059 w1073 w1090 w1093 w1113 w1126 w1133 w1142 w1153 w1161 w1175 w1198 w1208 w1215 w1227 w1239 w1249 w1256 w1277 w1286 w1291 w1300 w1309 w1318 w1329 w1340 w1349 w1360 w1371 w1381] -> w206
      tunnel: w204 -> [w956 w964 w972 w983 w993 w1007 w1014 w1025 w1038 w1046 w1053 w1066 w1085 w1092 w1104 w1125 w1132 w1141 w1152 w1160 w1172 w1197 w1205 w1214 w1226 w1238 w1248 w1255 w1278 w1287 w1290 w1297 w1306 w1315 w1330 w1341 w1344 w1361 w1372 w1382]
      tunnel: [w956 w964 w972 w983 w993 w1007 w1014 w1025 w1038 w1046 w1053 w1066 w1084 w1092 w1103 w1125 w1132 w1141 w1152 w1160 w1171 w1197 w1205 w1214 w1226 w1238 w1248 w1255 w1278 w1287 w1290 w1297 w1306 w1315 w1330 w1341 w1344 w1361 w1372 w1382] -> w203
      tunnel: w201 -> [w953 w963 w973 w984 w994 w1003 w1015 w1026 w1035 w1045 w1052 w1065 w1081 w1091 w1099 w1122 w1131 w1140 w1151 w1158 w1169 w1195 w1204 w1213 w1225 w1237 w1247 w1254 w1279 w1288 w1289 w1296 w1305 w1314 w1331 w1342 w1343 w1355 w1366 w1376]
      tunnel: [w953 w963 w973 w984 w994 w1003 w1015 w1026 w1035 w1045 w1052 w1065 w1081 w1091 w1099 w1122 w1131 w1140 w1151 w1158 w1168 w1195 w1204 w1213 w1225 w1237 w1247 w1254 w1279 w1288 w1289 w1296 w1305 w1314 w1331 w1342 w1343 w1355 w1364 w1375] -> w200
      tunnel: w198 -> [_ _ _ _ _ _ _ _ _ _ _ _ _ _ _ _ _ _ _ _ _ _ _ _ _ _ _ _ _ _ _ _ _ _ _ w1333 _ _ _ _]
      frame "Exit" {
        # ">>State Logic  >>"
        # ">>> Time cluster >>>"
        # ">>> Yaw >>>"
        # ">>> Stepper position >>>"
        # ">>> Encoders >>>"
        # ">>> Object detection >>>"
        # ">>> Ultrasonic Sensors Detect >>>"
        n62 = call "Imaq Dispose"("All Images? (No)"=TRUE, "Image"=w954) -> ()  [unwired: 4 in, 1 out]
      }
      frame "----Movement States----" {
        # ">>State Logic  >>"
        # ">>> Time cluster >>>"
        # ">>> Yaw >>>"
        # ">>> Stepper position >>>"
        # ">>> Encoders >>>"
        # ">>> Object detection >>>"
        # ">>> Ultrasonic Sensors Detect >>>"
      }
      frame "FORWARD" {
        # ">>> Time cluster >>>"
        # ">>> Yaw >>>"
        # ">>> Stepper position >>>"
        # ">>> Encoders >>>"
        # ">>> Object detection >>>"
        # ">>> Ultrasonic Sensors Detect >>>"
        n63 = Unbundle By Name(w972) -> ("Yaw"=w971:dbl)
        n64 = call "Motor Control NO PID AE Ver.vi"("Direction"=MOTOR_CONTROL_NO_PID_AE_DIRECTIONS_type_def."y-axis movement", "AE Mode"=MOTOR_CONTROL_NO_PID_AE_DATA_ENTRY_MODE_Type_def."Write to motors", "Speed"=0.5, "Yaw"=w971) -> ()  [unwired: 1 in, 2 out]
      }
      frame "LEFT" {
        # ">>State Logic  >>"
        # ">>> Time cluster >>>"
        # ">>> Yaw >>>"
        # ">>> Stepper position >>>"
        # ">>> Encoders >>>"
        # ">>> Object detection >>>"
        # ">>> Ultrasonic Sensors Detect >>>"
        n65 = Unbundle By Name(w983) -> ("Yaw"=w982:dbl)
        n66 = call "Motor Control NO PID AE Ver.vi"("Direction"=MOTOR_CONTROL_NO_PID_AE_DIRECTIONS_type_def."x-axis movement", "AE Mode"=MOTOR_CONTROL_NO_PID_AE_DATA_ENTRY_MODE_Type_def."Write to motors", "Speed"=-0.5, "Yaw"=w982) -> ()  [unwired: 1 in, 2 out]
      }
      frame "R-ACW" {
        n67 = call "Motor Control NO PID AE Ver.vi"("Direction"=MOTOR_CONTROL_NO_PID_AE_DIRECTIONS_type_def."Rotate", "AE Mode"=MOTOR_CONTROL_NO_PID_AE_DATA_ENTRY_MODE_Type_def."Write to motors", "Speed"=0.25) -> ()  [unwired: 2 in, 2 out]
      }
      frame "R-CW" {
        (unwired) -0.2 ("Speed")
        n68 = call "Motor Control NO PID AE Ver.vi"("Direction"=MOTOR_CONTROL_NO_PID_AE_DIRECTIONS_type_def."Rotate", "AE Mode"=MOTOR_CONTROL_NO_PID_AE_DATA_ENTRY_MODE_Type_def."Write to motors", "Speed"=-0.5) -> ()  [unwired: 2 in, 2 out]
      }
      frame "RIGHT" {
        n69 = Unbundle By Name(w1014) -> ("Yaw"=w1013:dbl)
        n70 = call "Motor Control NO PID AE Ver.vi"("Direction"=MOTOR_CONTROL_NO_PID_AE_DIRECTIONS_type_def."x-axis movement", "AE Mode"=MOTOR_CONTROL_NO_PID_AE_DATA_ENTRY_MODE_Type_def."Write to motors", "Speed"=0.5, "Yaw"=w1013) -> ()  [unwired: 1 in, 2 out]
      }
      frame "REVERSE" {
        n71 = Unbundle By Name(w1025) -> ("Yaw"=w1024:dbl)
        n72 = call "Motor Control NO PID AE Ver.vi"("Direction"=MOTOR_CONTROL_NO_PID_AE_DIRECTIONS_type_def."y-axis movement", "AE Mode"=MOTOR_CONTROL_NO_PID_AE_DATA_ENTRY_MODE_Type_def."Write to motors", "Speed"=-0.5, "Yaw"=w1024) -> ()  [unwired: 1 in, 2 out]
      }
      frame "STOP" {
        n73 = Wait (ms)(milliseconds to wait=u32 500) -> ()  [unwired: 1 out]
        n74 = call "Motor Control NO PID AE Ver.vi"("Direction"=MOTOR_CONTROL_NO_PID_AE_DIRECTIONS_type_def."Stop", "AE Mode"=MOTOR_CONTROL_NO_PID_AE_DATA_ENTRY_MODE_Type_def."Write to motors") -> ()  [unwired: 3 in, 2 out]
      }
      frame "----SENSOR READING---- " {
      }
      frame "READ ENCODERS" {
        # ">>> Time cluster >>>"
        # ">>> Yaw >>>"
        # ">>> Stepper position >>>"
        # ">>> Object detection >>>"
        # ">>> Current encoder distance >>>"
        # ">>> Ultrasonic Sensors Detect >>>"
        n75 = call "Motor Control NO PID AE Ver.vi"("AE Mode"=MOTOR_CONTROL_NO_PID_AE_DATA_ENTRY_MODE_Type_def."Read from Encoders") -> ("Speed & distance"=w1057:T2)  [unwired: 4 in, 1 out]
        n76 = Unbundle By Name(w1057) -> ("xDistance"=w1056:dbl, "yDistance"=w1055:dbl, "wDistance"=w1054:dbl)
        n77 = Bundle By Name(cluster=w1062, "xDistance"=w1056, "yDistance"=w1055, "wDistance"=w1054) -> (w1061:T15)
      }
      frame "READ ULTRASONIC" {
        (unwired) navX_type_def."Read Values" ("Mode")
        (unwired) MOTOR_CONTROL_NO_PID_Type_Def."Latch" ("Direction")
        # ">>> Ultrasonic Sensors Detect >>>"
        # ">>> Object detection >>>"
        # ">>> Encoders >>>"
        # ">>> Stepper position >>>"
        # ">>> Yaw >>>"
        n78 = call "Arduino Interfacing VI.vi"("AE Mode"=Arduino_Interfacing."Read From Arduino") -> ("Arduino Data"=w1071:T4)  [unwired: 3 in, 1 out]
        n79 = Unbundle By Name(w1071) -> ("PING A"=w1070:u8, "PING B"=w1069:u8, "PING C"=w1068:u8, "PING D"=w1067:u8)
        n80 = Bundle By Name(cluster=w1077, "PING_A"=w1070, "PING_B"=w1069, "PING_C"=w1068, "PING_D"=w1067) -> (w1078:T14)
      }
      frame "READ YAW" {
        # ">>> Time cluster >>>"
        # ">>> Yaw >>>"
        # ">>> Ultrasonic Sensors Detect >>>"
        # ">>> Object detection >>>"
        # ">>> Encoders >>>"
        # ">>> Stepper position >>>"
        n81 = call "navX reading VI.vi"("Mode"=navX_type_def."Read Values") -> ("NavX Readings"=w1080:T3)  [unwired: 2 in, 3 out]
        n82 = Unbundle By Name(w1080) -> ("Heading"=w1079:dbl)
        n83 = Unbundle By Name(w1080) -> ("Yaw"=w1083:dbl)
        n84 = Bundle By Name(cluster=w1085, "Yaw"=w1083, "Compass"=w1079) -> (w1084:T10)
      }
      frame "----SYSTEM MODES----" {
        (unwired) I2C_MASTER_Type_Def."Last State" ("Arduino Mode")
        # ">>> Object detection >>>"
        # ">>> Yaw >>>"
        # ">>> Ultrasonic Sensors Detect >>>"
        # ">>> Encoders >>>"
        # ">>> Stepper position >>>"
      }
      frame "INIT" {
        w1115 = u8 0
        w1116 = 0.0
        # ">>> Time cluster >>>"
        # ">>> Object detection >>>"
        # ">>> Yaw >>>"
        # ">>> Ultrasonic Sensors Detect >>>"
        # ">>> Encoders >>>"
        # ">>> Stepper position >>>"
        # ">>State Logic  >>"
        n85 = call "Arduino Interfacing VI.vi"("AE Mode"=Arduino_Interfacing."Initialize") -> ()  [unwired: 3 in, 2 out]
        n86 = call "FGV Bool.vi"("Init/Read/Write State"=States_for_Action_Engine."Initialize") -> ()  [unwired: 2 in, 2 out]
        n87 = call "Motor Control NO PID AE Ver.vi"("AE Mode"=MOTOR_CONTROL_NO_PID_AE_DATA_ENTRY_MODE_Type_def."Initialize") -> ()  [unwired: 4 in, 2 out]
        n88 = call "Elasped Timer.vi"("Action"=Elapsed_timer_control."Initialize") -> ()  [unwired: 7 in, 4 out]
        n89 = Bundle By Name(cluster=w1109, "Recognized Object"=FALSE, "Object X coordinate"=0.0, "Object Y coordinate"=0.0) -> (w1108:T13)
        n90 = Bundle By Name(cluster=w1114, "y Stepper Position"=u8 0, "z Stepper Position"=u8 0) -> (w1113:T11)
        n91 = Bundle By Name(cluster=w1118, "xDistance"=w1116, "yDistance"=w1116, "wDistance"=w1116) -> (w1117:T15)
        n92 = Bundle By Name(cluster=w1120, "PING_A"=w1115, "PING_B"=w1115, "PING_C"=w1115, "PING_D"=w1115) -> (w1121:T14)
        n93 = Bundle By Name(cluster=w1104, "Yaw"=0.0) -> (w1103:T10)
      }
      frame "ARDUINO - ULTRASONIC" {
        # ">>> Object detection >>>"
        # ">>> Yaw >>>"
        # ">>> Ultrasonic Sensors Detect >>>"
        # ">>> Encoders >>>"
        # ">>> Stepper position >>>"
        # ">>State Logic  >>"
        n94 = call "Arduino Interfacing VI.vi"("Data to Write"=I2C_MASTER_WRITE_NEW_Type_Def."Ultrasonic sensors", "AE Mode"=Arduino_Interfacing."Write to Arduino") -> ()  [unwired: 2 in, 2 out]
      }
      frame "NAVX CALIBRATE" {
        # ">>> Object detection >>>"
        # ">>> Yaw >>>"
        # ">>> Ultrasonic Sensors Detect >>>"
        # ">>> Encoders >>>"
        # ">>> Stepper position >>>"
        # ">>State Logic  >>"
        # "Adds a 15 second delay to the startup process \nfor the NavX to calibrate"
        n95 = Wait (ms)(milliseconds to wait=u32 5000) -> ()  [unwired: 1 out]
      }
      frame "NO ACTION", Default {
        (unwired) u8 0 ("y Stepper value")
        (unwired) TRUE ("Latch")
        (unwired) navX_type_def."Read Values" ("Mode")
        (unwired) MOTOR_CONTROL_NO_PID_Type_Def."Latch" ("Direction")
        # ">>> Object detection >>>"
        # ">>> Yaw >>>"
        # ">>> Ultrasonic Sensors Detect >>>"
        # ">>> Encoders >>>"
        # ">>> Stepper position >>>"
        # ">>State Logic  >>"
        n96 = case shown="4" w1145 {
          tunnel: [0 100] -> w1147
          frame 1, Default {
          }
          frame 4 {
          }
        }
      }
      frame "----RESET CASES----" {
        (unwired) I2C_MASTER_Type_Def."Last State" ("Arduino Mode")
        # ">>> Object detection >>>"
        # ">>> Yaw >>>"
        # ">>> Ultrasonic Sensors Detect >>>"
        # ">>> Encoders >>>"
        # ">>> Stepper position >>>"
        # ">>State Logic  >>"
      }
      frame "RESET ENCODERS" {
        # ">>> Object detection >>>"
        # ">>> Yaw >>>"
        # ">>> Ultrasonic Sensors Detect >>>"
        # ">>> Encoders >>>"
        # ">>> Stepper position >>>"
        # ">>State Logic  >>"
        n97 = call "Motor Control NO PID AE Ver.vi"("AE Mode"=MOTOR_CONTROL_NO_PID_AE_DATA_ENTRY_MODE_Type_def."Reset Encoders") -> ()  [unwired: 4 in, 2 out]
      }
      frame "RESET FLAGS" {
        (unwired) I2C_MASTER_Type_Def."Last State" ("Arduino Mode")
        # "Resets any software variables\nand/or non-critical states"
        n98 = Wait (ms)(milliseconds to wait=u32 20) -> ()  [unwired: 1 out]
        n99 = Bundle By Name(cluster=w1169, "Time up flag"=FALSE, "SET TIME TO CHECK"=0.0) -> (w1168:T9)
        n100 = Bundle By Name(cluster=w1186, "Recognized Object"=FALSE, "Object X coordinate"=0.0, "Object Y coordinate"=0.0) -> (w1185:T13)
        n101 = Bundle By Name(cluster=w1176, "y Stepper Position"=u8 0, "z Stepper Position"=u8 0) -> (w1175:T11)
        n102 = Bundle By Name(cluster=w1181, "xDistance"=0.0, "yDistance"=0.0, "wDistance"=0.0) -> (w1180:T15)
        n103 = Bundle By Name(cluster=w1193, "PING_A"=u8 0, "PING_B"=u8 0, "PING_C"=u8 0, "PING_D"=u8 0) -> (w1192:T14)
        n104 = Bundle By Name(cluster=w1172, "Yaw"=0.0) -> (w1171:T10)
      }
      frame "RESET YAW" {
        n105 = Wait (ms)(milliseconds to wait=u32 100) -> ()  [unwired: 1 out]
        n106 = call "navX reading VI.vi"("Mode"=navX_type_def."Zero Yaw") -> ()  [unwired: 2 in, 4 out]
      }
      frame "RESET ARM" {
        n107 = call "Arduino Interfacing VI.vi"("Data to Write"=I2C_MASTER_WRITE_NEW_Type_Def."Soft Reset", "AE Mode"=Arduino_Interfacing."Write to Arduino") -> ()  [unwired: 2 in, 2 out]
      }
      frame "--------CAM STATES-------" {
      }
      frame "OPEN LOG CAM" {
        n108 = call "Webcam AE.vi"("Session In"=T29 "cam0", "Camera states"=Webcam_AE."Initialize Camera") -> ("error out"=w1222:errorcluster, "Session Out"=w1221:T29)  [unwired: 1 in, 1 out]
        n109 = call "Webcam AE.vi"("error in (no error)"=w1222, "Session In"=w1221, "Camera states"=Webcam_AE."Open Camera") -> ()  [unwired: 3 out]
      }
      frame "OPEN LIFE CAM" {
        n110 = call "Webcam AE.vi"("Session In"=T29 "cam1", "Camera states"=Webcam_AE."Initialize Camera") -> ("error out"=w1234:errorcluster, "Session Out"=w1233:T29)  [unwired: 1 in, 1 out]
        n111 = call "Webcam AE.vi"("error in (no error)"=w1234, "Session In"=w1233, "Camera states"=Webcam_AE."Open Camera") -> ()  [unwired: 3 out]
      }
      frame "CAM ACQ" {
        # ">>State Logic  >>"
        # ">>> Time cluster >>>"
        # ">>> Yaw >>>"
        # ">>> Stepper position >>>"
        # ">>> Encoders >>>"
        # ">>> Object detection >>>"
        # ">>> Ultrasonic Sensors Detect >>>"
        n112 = call "Webcam AE.vi"("error in (no error)"=w1244, "Camera states"=Webcam_AE."Continuous Acquisition") -> ()  [unwired: 1 in, 3 out]
      }
      frame "CAM CLOSE" {
        # ">>State Logic  >>"
        # ">>> Time cluster >>>"
        # ">>> Yaw >>>"
        # ">>> Stepper position >>>"
        # ">>> Encoders >>>"
        # ">>> Object detection >>>"
        # ">>> Ultrasonic Sensors Detect >>>"
        n113 = call "Webcam AE.vi"("Camera states"=Webcam_AE."Close Camera") -> ()  [unwired: 2 in, 3 out]
      }
      frame "PROCESS IMAGE" {
        # ">>State Logic  >>"
        # ">>> Time cluster >>>"
        # ">>> Yaw >>>"
        # ">>> Stepper position >>>"
        # ">>> Encoders >>>"
        # ">>> Object detection >>>"
        # ">>> Ultrasonic Sensors Detect >>>"
        n114 = call "Webcam AE.vi"("error in (no error)"=w1272, "Camera states"=Webcam_AE."Retrieve Image") -> ("error out"=w1268:errorcluster, "Image Out"=w1271:T23)  [unwired: 1 in, 1 out]
        n115 = call "Object Detection SubVI.vi"("Error In"=w1268, "Mode"="Object recognition mode", "Image Dest"=w1270, "Image in"=w1271) -> ("Object Center Coordinates"=w1265:cluster{"x":sgl, "y":sgl}, "Object detection cluster"=w1261:T1)  [unwired: 2 out]
        "Object detection cluster" <- w1261
        "Object Center Coordinates" <- w1265
        n116 = Unbundle By Name(w1261) -> ("Object detected?"=w1262:bool)
        n117 = Unbundle By Name(w1265) -> ("x"=w1264:sgl, "y"=w1263:sgl)
        n118 = Bundle By Name(cluster=w1267, "Recognized Object"=w1262, "Object X coordinate"=w1264, "Object Y coordinate"=w1263) -> (w1266:T13)
      }
      frame "DISPOSE BUFFERS" {
        # ">>State Logic  >>"
        # ">>> Time cluster >>>"
        # ">>> Yaw >>>"
        # ">>> Stepper position >>>"
        # ">>> Encoders >>>"
        # ">>> Object detection >>>"
        # ">>> Ultrasonic Sensors Detect >>>"
        n119 = call "Webcam AE.vi"("error in (no error)"=w1281, "Camera states"=Webcam_AE."Dispose Image Buffers") -> ()  [unwired: 1 in, 3 out]
      }
      frame "-----ARM ACTIONS-----" {
      }
      frame "CLOSE CLAW" {
        n120 = call "Arduino Interfacing VI.vi"("Data to Write"=I2C_MASTER_WRITE_NEW_Type_Def."Close Claw", "AE Mode"=Arduino_Interfacing."Write to Arduino") -> ()  [unwired: 2 in, 2 out]
      }
      frame "OPEN CLAW" {
        n121 = call "Arduino Interfacing VI.vi"("Data to Write"=I2C_MASTER_WRITE_NEW_Type_Def."Open Claw", "AE Mode"=Arduino_Interfacing."Write to Arduino") -> ()  [unwired: 2 in, 2 out]
      }
      frame "Z STEPPER CAM HEIGHT" {
        n122 = call "Arduino Interfacing VI.vi"("Data to Write"=I2C_MASTER_WRITE_NEW_Type_Def."zStepper 8k", "AE Mode"=Arduino_Interfacing."Write to Arduino") -> ()  [unwired: 2 in, 2 out]
      }
      frame "Z STEPPER GRAB HEIGHT" {
        # ">>State Logic  >>"
        # ">>> Time cluster >>>"
        # ">>> Yaw >>>"
        # ">>> Stepper position >>>"
        # ">>> Encoders >>>"
        # ">>> Object detection >>>"
        # ">>> Ultrasonic Sensors Detect >>>"
        n123 = call "Arduino Interfacing VI.vi"("Data to Write"=I2C_MASTER_WRITE_NEW_Type_Def."zStepper 100", "AE Mode"=Arduino_Interfacing."Write to Arduino") -> ()  [unwired: 2 in, 2 out]
      }
      frame "Y STEPPER CONTROL" {
        # ">>State Logic  >>"
        # ">>> yStepper command>>>"
        # ">>> Time cluster >>>"
        # ">>> Yaw >>>"
        # ">>> Stepper position >>>"
        # ">>> Encoders >>>"
        # ">>> Object detection >>>"
        # ">>> Ultrasonic Sensors Detect >>>"
        n124 = Unbundle By Name(w1333) -> ("yStepper desired"=w1332:u8)
        n125 = call "Arduino Interfacing VI.vi"("y Stepper value"=w1332, "Data to Write"=I2C_MASTER_WRITE_NEW_Type_Def."yStepper control", "AE Mode"=Arduino_Interfacing."Write to Arduino") -> ()  [unwired: 1 in, 2 out]
      }
      frame "READ STEPPER VALUES" {
        # ">>State Logic  >>"
        # ">>> Time cluster >>>"
        # ">>> Yaw >>>"
        # ">>> Stepper position >>>"
        # ">>> Encoders >>>"
        # ">>> Object detection >>>"
        # ">>> Ultrasonic Sensors Detect >>>"
        n126 = call "Arduino Interfacing VI.vi"("AE Mode"=Arduino_Interfacing."Read From Arduino") -> ("Arduino Data"=w1347:T4)  [unwired: 3 in, 1 out]
        n127 = Unbundle By Name(w1347) -> ("y Stepper Position"=w1346:u8, "z Stepper Position"=w1345:u8)
        n128 = Bundle By Name(cluster=w1350, "y Stepper Position"=w1346, "z Stepper Position"=w1345) -> (w1349:T11)
      }
      frame " -----TIMING-----" {
        # ">>State Logic  >>"
        # ">>> Time cluster >>>"
        # ">>> Yaw >>>"
        # ">>> Stepper position >>>"
        # ">>> Encoders >>>"
        # ">>> Object detection >>>"
        # ">>> Ultrasonic Sensors Detect >>>"
      }
      frame "SET TIMER" {
        # ">>State Logic  >>"
        # ">>> Time cluster >>>"
        # ">>> Yaw >>>"
        # ">>> Stepper position >>>"
        # ">>> Encoders >>>"
        # ">>> Object detection >>>"
        # ">>> Ultrasonic Sensors Detect >>>"
        n129 = call "Elasped Timer.vi"("Time Setting"=5.0, "Action"=Elapsed_timer_control."Initialize") -> ()  [unwired: 6 in, 4 out]
        n130 = Bundle By Name(cluster=w1366, "Time up flag"=FALSE) -> (w1364:T9)
      }
      frame "START TIMER" {
        # ">>State Logic  >>"
        # ">>> Time cluster >>>"
        # ">>> Yaw >>>"
        # ">>> Stepper position >>>"
        # ">>> Encoders >>>"
        # ">>> Object detection >>>"
        # ">>> Ultrasonic Sensors Detect >>>"
        n131 = call "Elasped Timer.vi"("Action"=Elapsed_timer_control."Start") -> ("Time Out?!"=w1373:bool)  [unwired: 7 in, 3 out]
        n132 = Bundle By Name(cluster=w1376, "Time up flag"=w1373) -> (w1375:T9)
      }
    }
    "State Logic" <- w222
    n133 = local read "TASK ENABLE"() -> (w216:bool)
    n134 = Not(x=w216) -> (.not. x?=w215:bool)
    n135 = case shown="True" w223 {
      tunnel: w227 -> [w250 w281]
      tunnel: w231 -> [w246 w283]
      tunnel: [w250 w281] -> w236
      tunnel: [w246 w284] -> w235
      tunnel: w232 -> [_ w279]
      tunnel: w234 -> [_ w280]
      tunnel: w229 -> [w249 w286]
      tunnel: [w249 w286] -> w228
      tunnel: "STOP TASK" -> [_ w269]
      tunnel: w222 -> [w248 w285]
      tunnel: [w248 w282] -> w221
      tunnel: w218 -> [w247 w275]
      tunnel: [w247 w275] -> w217
      tunnel: w215 -> [_ w270]
      tunnel: [w245 w267] -> w214
      tunnel: w213 -> [w245 w266]
      tunnel: w209 -> [w244 w263]
      tunnel: [w244 w263] -> w208
      tunnel: w206 -> [w243 w259]
      tunnel: [w243 w259] -> w205
      tunnel: w203 -> [w242 w257]
      tunnel: [w242 w257] -> w202
      tunnel: w200 -> [w241 w255]
      tunnel: [w241 w255] -> w199
      tunnel: w198 -> [w240 w254]
      tunnel: [w240 w253] -> w197
      tunnel: [_ w251] -> w196
      frame False {
        # ">>> yStepper command>>>"
        # ">>> Time cluster >>>"
        # ">>> Yaw >>>"
        # ">>> Stepper position >>>"
        # ">>> Encoders >>>"
        # ">>> Object detection >>>"
        # ">>> Ultrasonic Sensors Detect >>>"
        # ">>> Time cluster >>>"
        # ">>> Yaw >>>"
        # ">>> Stepper position >>>"
        # ">>> Encoders >>>"
        # ">>> Object detection >>>"
        # ">>> Ultrasonic Sensors Detect >>>"
      }
      frame True {
        # ">>State Logic Queue Reference >>"
        # ">>Timeout>>"
        # ">>> yStepper command>>>"
        # ">>> Time cluster >>>"
        # ">>> Object detection >>>"
        # ">>> Yaw >>>"
        # ">>> Ultrasonic Sensors Detect >>>"
        # ">>> Encoders >>>"
        # ">>> Stepper position >>>"
        # ">>State Logic  >>"
        # ">>True Stop Next State >>"
        # ">>Action Queue>>"
        # ">> Manual override >>"
        # ">>> Time cluster >>>"
        # ">>> Yaw >>>"
        # ">>> Stepper position >>>"
        # ">>> Encoders >>>"
        # ">>> Object detection >>>"
        # ">>> Ultrasonic Sensors Detect >>>"
        # ">>Action Queue>>"
        # ">>State Logic Queue Reference >>"
        n136 = Or(x=w269, y=w270) -> (x .or. y?=w268:bool)
        n137 = Unbundle By Name(w257) -> ("Yaw"=w258:dbl, "Compass"=w252:dbl)
        n138 = Unbundle By Name(w255) -> ("Time up flag"=w256:bool)
        "Time up flag" <- w256
        n139 = Unbundle By Name(w259) -> ("y Stepper Position"=w261:u8, "z Stepper Position"=w260:u8)
        n140 = Unbundle By Name(w275) -> ("xDistance"=w272:dbl, "yDistance"=w273:dbl, "wDistance"=w274:dbl)
        n141 = Unbundle By Name(w263) -> ("Recognized Object"=w262:bool, "Object X coordinate"=w265:dbl, "Object Y coordinate"=w264:dbl)
        n142 = Unbundle By Name(w286) -> ("PING_A"=w278:u8, "PING_B"=w277:u8, "PING_C"=w276:u8, "PING_D"=w271:u8)
        n143 = case shown="3" w285 {
          tunnel: [w289 w295 w307 w316 w376 w389 w426 w473 w515 w567 w613 w652 w711 w755 w794 w839 w882 w924] -> w284
          tunnel: w283 -> [w289 w298 w308 w319 w378 w390 w427 w474 w521 w560 w616 w659 w701 w758 w800 w838 w877 w915]
          tunnel: [State_Type_Definitions."Idle" ("Enum") State_Type_Definitions."Idle" ("Enum") w303 w318 State_Type_Definitions."Shutdown" ("Enum") w391 w429 w472 w516 w566 w614 w654 w710 w756 w801 w840 w883 w916] -> w282
          tunnel: w281 -> [_ _ w306 w322 _ w396 w439 w481 w520 w564 w617 w658 w708 w753 w799 w836 w880 w923]
          tunnel: w280 -> [_ _ _ w321 _ w395 w438 w480 w519 w563 w610 w657 w707 w752 w798 w835 w879 w921]
          tunnel: w279 -> [_ _ w305 w317 _ w394 w437 w479 w518 w562 w609 w656 w709 w754 w797 w834 w878 w922]
          tunnel: w268 -> [_ _ _ _ _ w388 w428 w476 w514 w565 w615 w660 w702 w759 w795 w837 w881 w919]
          tunnel: w278 -> [_ _ _ _ _ _ _ _ _ _ _ _ _ _ _ _ _ _]
          tunnel: w277 -> [_ _ _ _ _ _ w435 _ _ w556 w598 w650 _ w745 _ _ _ _]
          tunnel: w276 -> [_ _ _ _ _ _ w434 _ _ w557 w599 w651 _ w746 _ _ _ _]
          tunnel: w274 -> [_ _ _ _ _ _ _ w478 _ _ _ _ _ _ _ _ _ _]
          tunnel: w273 -> [_ _ _ _ _ w387 _ _ _ _ _ w655 _ _ _ _ _ _]
          tunnel: w272 -> [_ _ _ _ _ _ _ _ _ _ w604 _ _ _ _ _ _ _]
          tunnel: w271 -> [_ _ _ _ _ _ _ _ _ _ _ _ _ _ _ _ _ _]
          tunnel: [State_Type_Definitions."Idle" ("Enum") State_Type_Definitions."Idle" ("Enum") State_Type_Definitions."Idle" ("Enum") State_Type_Definitions."Idle" ("Enum") State_Type_Definitions."Shutdown" ("Enum") w384 w425 w469 w513 w559 w612 w653 w712 w757 w793 w841 w884 w917] -> w267
          tunnel: w266 -> [_ _ w303 _ _ _ _ _ _ _ _ _ _ _ _ _ _ _]
          tunnel: w262 -> [_ _ _ _ _ _ _ _ _ _ _ _ _ _ _ w831 _ w918]
          tunnel: w265 -> [_ _ _ _ _ _ _ _ _ _ _ _ _ _ _ _ _ _]
          tunnel: w264 -> [_ _ _ _ _ _ _ _ _ _ _ _ _ _ _ _ _ _]
          tunnel: w261 -> [_ _ _ _ _ _ _ _ _ _ _ _ _ _ _ _ _ _]
          tunnel: w260 -> [_ _ _ _ _ _ _ _ w511 _ _ _ w705 _ _ _ w876 _]
          tunnel: w258 -> [_ _ _ _ _ _ _ _ _ _ _ _ _ _ _ _ _ _]
          tunnel: w256 -> [_ _ _ _ _ _ _ _ _ _ _ _ _ _ w791 _ _ _]
          tunnel: w254 -> [w287 w293 w302 w314 w374 w383 w424 w468 w512 w558 w608 w649 w700 w750 w792 w832 w873 w914]
          tunnel: [w287 w292 w302 w314 w374 w383 w424 w468 w512 w558 w608 w649 w700 w750 w792 w832 w873 w914] -> w253
          tunnel: w252 -> [_ _ _ _ _ _ _ _ _ _ _ _ _ _ _ _ _ _]
          tunnel: [_ _ _ TRUE _ _ _ _ _ _ _ _ _ _ _ _ _ _] -> w251
          frame 0 {
            # ">>> yStepper command>>>"
          }
          frame 1 {
            # ">>> yStepper command>>>"
            n144 = for {
              shift-right: [w301] -> w295
              shift-left: w298 -> [w300]
              tunnel: string[] ["INIT", "RESET ARM", "RESET FLAGS", "RESET YAW", "NAVX CALIBRATE"] -> [w299] mode=indexing
              n145 = Enqueue Element(queue=w300, element=w299) -> (queue out=w301:refnum<queue>)  [unwired: 2 in, 2 out]
            }
            n146 = Bundle By Name(cluster=w293, "yStepper desired"=u8 0) -> (w292:T8)
          }
          frame 3 {
            # ">>> yStepper command>>>"
            n147 = Flush Queue(queue=w306, error in (no error)=w305) -> ()  [unwired: 3 out]
            n148 = for {
              shift-right: [w312] -> w307
              shift-left: w308 -> [w311]
              tunnel: string[] ["STOP", "RESET ENCODERS", "RESET YAW", "RESET ARM", "RESET FLAGS", "DISPOSE BUFFERS", "CAM CLOSE"] -> [w310] mode=indexing
              n149 = Enqueue Element(queue=w311, element=w310) -> (queue out=w312:refnum<queue>)  [unwired: 2 in, 2 out]
            }
          }
          frame 4, Default {
            (unwired) TRUE ("Green LED")
            # ">>> yStepper command>>>"
            n150 = Dequeue Element(queue=w322, timeout in ms (-1)=w321, error in (no error)=w317) -> (element=w320:T7)  [unwired: 3 out]
            n151 = case shown="\"Start Task 4\"" w320 {
              tunnel: [w324 w331 w338 w345 w352 w359 w366 w368] -> w316
              tunnel: w319 -> [w325 w332 w339 w346 w353 w360 w366 w369]
              tunnel: [State_Type_Definitions."Task 1" ("Enum") State_Type_Definitions."Task 2" ("Enum") State_Type_Definitions."Task 3" ("Enum") State_Type_Definitions."Task 4_A" ("Enum") State_Type_Definitions."Task 5_A" ("Enum") State_Type_Definitions."Task 6_A" ("Enum") State_Type_Definitions."Idle" ("Enum") State_Type_Definitions."Shutdown" ("Enum")] -> w318
              frame "Start Task 1" {
                n152 = for {
                  shift-right: [w329] -> w324
                  shift-left: w325 -> [w328]
                  tunnel: string[] ["RESET ENCODERS", "RESET YAW", "FORWARD", "READ ENCODERS"] -> [w327] mode=indexing
                  n153 = Enqueue Element(queue=w328, element=w327) -> (queue out=w329:refnum<queue>)  [unwired: 2 in, 2 out]
                }
              }
              frame "Start Task 2" {
                n154 = for {
                  shift-right: [w336] -> w331
                  shift-left: w332 -> [w335]
                  tunnel: string[] ["RESET ENCODERS", "RESET YAW", "READ ULTRASONIC", "ARDUINO - ULTRASONIC"] -> [w334] mode=indexing
                  n155 = Enqueue Element(queue=w335, element=w334) -> (queue out=w336:refnum<queue>)  [unwired: 2 in, 2 out]
                }
              }
              frame "Start Task 3" {
                n156 = for {
                  shift-right: [w343] -> w338
                  shift-left: w339 -> [w342]
                  tunnel: string[] ["RESET ENCODERS", "READ ENCODERS", "R-ACW"] -> [w341] mode=indexing
                  n157 = Enqueue Element(queue=w342, element=w341) -> (queue out=w343:refnum<queue>)  [unwired: 2 in, 2 out]
                }
              }
              frame "Start Task 4" {
                n158 = for {
                  shift-right: [w350] -> w345
                  shift-left: w346 -> [w349]
                  tunnel: string[] ["RESET YAW", "RESET ENCODERS", "RESET ARM", "RESET FLAGS", "", ""] -> [w348] mode=indexing
                  n159 = Enqueue Element(queue=w349, element=w348) -> (queue out=w350:refnum<queue>)  [unwired: 2 in, 2 out]
                }
              }
              frame "Start Task 5" {
                n160 = for {
                  shift-right: [w357] -> w352
                  shift-left: w353 -> [w356]
                  tunnel: string[] ["RESET YAW", "RESET ENCODERS", "READ STEPPER VALUES", "Z STEPPER CAM HEIGHT", "", ""] -> [w355] mode=indexing
                  n161 = Enqueue Element(queue=w356, element=w355) -> (queue out=w357:refnum<queue>)  [unwired: 2 in, 2 out]
                }
              }
              frame "Start Task 6" {
                n162 = for {
                  shift-right: [w364] -> w359
                  shift-left: w360 -> [w363]
                  tunnel: string[] ["OPEN LOG CAM ", "", "", "", "", ""] -> [w362] mode=indexing
                  n163 = Enqueue Element(queue=w363, element=w362) -> (queue out=w364:refnum<queue>)  [unwired: 2 in, 2 out]
                }
              }
              frame "None", Default {
              }
              frame "Exit" {
                n164 = for {
                  shift-right: [w373] -> w368
                  shift-left: w369 -> [w372]
                  tunnel: string[] ["STOP", "RESET ENCODERS", "RESET YAW", "EXIT"] -> [w371] mode=indexing
                  n165 = Enqueue Element(queue=w372, element=w371) -> (queue out=w373:refnum<queue>)  [unwired: 2 in, 2 out]
                }
              }
            }
          }
          frame 5 {
            # ">>> yStepper command>>>"
            n166 = for {
              shift-right: [w382] -> w376
              shift-left: w378 -> [w381]
              tunnel: string[] ["INIT", "RESET ENCODERS", "RESET FLAGS", "CAM CLOSE", "DISPOSE BUFFERS", "EXIT", ""] -> [w380] mode=indexing
              n167 = Enqueue Element(queue=w381, element=w380) -> (queue out=w382:refnum<queue>)  [unwired: 2 in, 2 out]
            }
          }
          frame 6 {
            # ">>> yStepper command>>>"
            # "Use 250"
            n168 = Dequeue Element(queue=w396, timeout in ms (-1)=w395, error in (no error)=w394) -> (element=w393:T7)  [unwired: 3 out]
            n169 = Greater?(x=w387, y=250.0) -> (0:w385:bool)
            n170 = Or(x=w385, y=w388) -> (x .or. y?=w392:bool)
            n171 = case shown="\"None\", Default" w393 {
              tunnel: w392 -> [w399 _]
              tunnel: [w403 State_Type_Definitions."True Stop" ("Enum")] -> w391
              tunnel: w390 -> [w400 w418]
              tunnel: [w398 w417] -> w389
              tunnel: [State_Type_Definitions."Idle" ("Enum") State_Type_Definitions."Shutdown" ("Enum")] -> w384
              frame "None", Default {
                n172 = case shown="True" w399 {
                  tunnel: w400 -> [w406 w412]
                  tunnel: [w405 w410] -> w398
                  frame False {
                    n173 = for {
                      shift-right: [w408] -> w405
                      shift-left: w406 -> [w409]
                      tunnel: string[] ["READ ENCODERS", "READ YAW", "FORWARD"] ("element") -> [w407] mode=indexing
                      n174 = Enqueue Element(queue=w409, element=w407) -> (queue out=w408:refnum<queue>)  [unwired: 2 in, 2 out]
                    }
                  }
                  frame True {
                    n175 = for {
                      shift-right: [w414] -> w410
                      shift-left: w412 -> [w415]
                      tunnel: string[] ["RESET YAW", "RESET ENCODERS", "STOP", ""] -> [w413] mode=indexing
                      n176 = Enqueue Element(queue=w415, element=w413) -> (queue out=w414:refnum<queue>)  [unwired: 2 in, 2 out]
                    }
                  }
                }
                n177 = Select(t=State_Type_Definitions."True Stop" ("Enum"), s=w399, f=State_Type_Definitions."Task 1" ("Enum")) -> (s? t:f=w403:u16)
              }
              frame "Exit" {
                n178 = for {
                  shift-right: [w422] -> w417
                  shift-left: w418 -> [w423]
                  tunnel: string[] ["STOP", "RESET ENCODERS", "RESET YAW", ""] -> [w421] mode=indexing
                  n179 = Enqueue Element(queue=w423, element=w421) -> (queue out=w422:refnum<queue>)  [unwired: 2 in, 2 out]
                }
              }
            }
          }
          frame 7 {
            w433 = u8 30 ("y")
            # ">>> yStepper command>>>"
            # ">>Object detected>>"
            n180 = Dequeue Element(queue=w439, timeout in ms (-1)=w438, error in (no error)=w437) -> (element=w436:T7)  [unwired: 3 out]
            n181 = Less?(x=w435, y=w433) -> (x < y?=w432:bool)
            n182 = Less?(x=w434, y=w433) -> (x < y?=w431:bool)
            n183 = Or(x=w432, y=w431) -> (x .or. y?=w430:bool)
            "Obstacle detected" <- w430
            n184 = case shown="\"None\", Default" w436 {
              tunnel: w430 -> [w443 _]
              tunnel: [w445 State_Type_Definitions."True Stop" ("Enum")] -> w429
              tunnel: w428 -> [w444 _]
              tunnel: w427 -> [w442 w462]
              tunnel: [w441 w463] -> w426
              tunnel: [State_Type_Definitions."Idle" ("Enum") State_Type_Definitions."Shutdown" ("Enum")] -> w425
              frame "None", Default {
                n185 = case shown="True" w443 {
                  tunnel: w442 -> [w449 w456]
                  tunnel: [w450 w455] -> w441
                  frame False {
                    n186 = for {
                      tunnel: string[] ["READ ULTRASONIC", "STOP"] ("element") -> [w451] mode=indexing
                      shift-right: [w453] -> w450
                      shift-left: w449 -> [w452]
                      n187 = Enqueue Element(queue=w452, element=w451) -> (queue out=w453:refnum<queue>)  [unwired: 2 in, 2 out]
                    }
                  }
                  frame True {
                    n188 = for {
                      shift-right: [w458] -> w455
                      shift-left: w456 -> [w459]
                      tunnel: string[] ["REVERSE", "READ ULTRASONIC", "READ YAW"] -> [w457] mode=indexing
                      n189 = Enqueue Element(queue=w459, element=w457) -> (queue out=w458:refnum<queue>)  [unwired: 2 in, 2 out]
                    }
                  }
                }
                n190 = Select(t=State_Type_Definitions."True Stop" ("Enum"), s=w444, f=State_Type_Definitions."Task 2" ("Enum")) -> (s? t:f=w445:u16)
              }
              frame "Exit" {
                n191 = for {
                  shift-right: [w466] -> w463
                  shift-left: w462 -> [w467]
                  tunnel: string[] ["STOP", "RESET ENCODERS", "RESET YAW", "ARDUINO MODE 0"] -> [w465] mode=indexing
                  n192 = Enqueue Element(queue=w467, element=w465) -> (queue out=w466:refnum<queue>)  [unwired: 2 in, 2 out]
                }
              }
            }
          }
          frame 11 {
            # ">>> yStepper command>>>"
            n193 = Dequeue Element(queue=w481, timeout in ms (-1)=w480, error in (no error)=w479) -> (element=w470:T7)  [unwired: 3 out]
            n194 = Greater?(x=w478, y=100.0) -> (0:w475:bool)
            n195 = Or(x=w475, y=w476) -> (x .or. y?=w471:bool)
            n196 = case shown="\"Exit\"" w470 {
              tunnel: w471 -> [w484 _]
              tunnel: [w488 State_Type_Definitions."True Stop" ("Enum")] -> w472
              tunnel: w474 -> [w485 w504]
              tunnel: [w483 w503] -> w473
              tunnel: [State_Type_Definitions."Idle" ("Enum") State_Type_Definitions."Shutdown" ("Enum")] -> w469
              frame "None", Default {
                n197 = case shown="False" w484 {
                  tunnel: w485 -> [w491 w497]
                  tunnel: [w490 w495] -> w483
                  frame False {
                    n198 = for {
                      shift-right: [w493] -> w490
                      shift-left: w491 -> [w494]
                      tunnel: string[] ["READ ENCODERS", "R-ACW"] ("element") -> [w492] mode=indexing
                      n199 = Enqueue Element(queue=w494, element=w492) -> (queue out=w493:refnum<queue>)  [unwired: 2 in, 2 out]
                    }
                  }
                  frame True {
                    n200 = for {
                      shift-right: [w499] -> w495
                      shift-left: w497 -> [w500]
                      tunnel: string[] ["RESET YAW", "RESET ENCODERS", "STOP", "ARDUINO MODE 0"] -> [w498] mode=indexing
                      n201 = Enqueue Element(queue=w500, element=w498) -> (queue out=w499:refnum<queue>)  [unwired: 2 in, 2 out]
                    }
                  }
                }
                n202 = Select(t=State_Type_Definitions."True Stop" ("Enum"), s=w484, f=State_Type_Definitions."Task 3" ("Enum")) -> (s? t:f=w488:T6)
              }
              frame "Exit" {
                n203 = for {
                  shift-right: [w507] -> w503
                  shift-left: w504 -> [w508]
                  tunnel: string[] ["STOP", "RESET ENCODERS", "RESET YAW", ""] -> [w506] mode=indexing
                  n204 = Enqueue Element(queue=w508, element=w506) -> (queue out=w507:refnum<queue>)  [unwired: 2 in, 2 out]
                }
              }
            }
          }
          frame 12 {
            # ">> Stepper height reeached >>"
            # ">>> yStepper command>>>"
            # ">> Manual override >>"
            n205 = Dequeue Element(queue=w520, timeout in ms (-1)=w519, error in (no error)=w518) -> (element=w517:T7)  [unwired: 3 out]
            n206 = Equal?(x=w511, y=u8 80) -> (x = y?=w509:bool)
            n207 = case shown="\"None\", Default" w517 {
              tunnel: [w532 State_Type_Definitions."True Stop" ("Enum")] -> w516
              tunnel: [w530 w547] -> w515
              tunnel: w521 -> [w529 _]
              tunnel: w514 -> [w523 _]
              tunnel: [State_Type_Definitions."Idle" ("Enum") State_Type_Definitions."Shutdown" ("Enum")] -> w513
              tunnel: w509 -> [w522 _]
              frame "None", Default {
                # ">> WIill proceed to part ii if not manual override >>"
                # ">>If ENABLE or Trigger is set to true>>"
                n208 = Or(x=w522, y=w523) -> (x .or. y?=w524:bool)
                n209 = case shown="True" w522 {
                  tunnel: [w535 w541] -> w530
                  tunnel: w529 -> [w534 w540]
                  frame False {
                    n210 = for {
                      shift-right: [w537] -> w535
                      shift-left: w534 -> [w538]
                      tunnel: string[] ["Z STEPPER CAM HEIGHT", "READ STEPPER VALUES"] ("element") -> [w536] mode=indexing
                      n211 = Enqueue Element(queue=w538, element=w536) -> (queue out=w537:refnum<queue>)  [unwired: 2 in, 2 out]
                    }
                  }
                  frame True {
                    n212 = for {
                      shift-right: [w543] -> w541
                      shift-left: w540 -> [w544]
                      tunnel: string[] ["ARDUINO - ULTRASONIC", "READ ULTRASONIC", "FORWARD", "", "", ""] -> [w542] mode=indexing
                      n213 = Enqueue Element(queue=w544, element=w542) -> (queue out=w543:refnum<queue>)  [unwired: 2 in, 2 out]
                    }
                  }
                }
                n214 = Select(t=State_Type_Definitions."True Stop" ("Enum"), s=w523, f=State_Type_Definitions."Task 4_B" ("Enum")) -> (s? t:f=w526:T6)
                n215 = Select(t=w526, s=w524, f=State_Type_Definitions."Task 4_A" ("Enum")) -> (s? t:f=w532:T6)
              }
              frame "Exit" {
                n216 = for {
                  shift-right: [w550] -> w547
                  shift-left: _ -> [w551]
                  tunnel: string[] ["STOP", "RESET ENCODERS", "RESET YAW", ""] -> [w549] mode=indexing
                  n217 = Enqueue Element(queue=w551, element=w549) -> (queue out=w550:refnum<queue>)  [unwired: 2 in, 2 out]
                }
              }
            }
          }
          frame 13 {
            w555 = u8 10
            # ">> Path blocked >>"
            # ">>> yStepper command>>>"
            # ">> Manual override >>"
            n218 = Dequeue Element(queue=w564, timeout in ms (-1)=w563, error in (no error)=w562) -> (element=w561:T7)  [unwired: 3 out]
            n219 = Less?(x=w557, y=w555) -> (x < y?=w552:bool)
            n220 = Less?(x=w556, y=w555) -> (x < y?=w553:bool)
            n221 = And(x=w553, y=w552) -> (x .and. y?=w554:bool)
            n222 = case shown="\"None\", Default" w561 {
              tunnel: [w578 State_Type_Definitions."True Stop" ("Enum")] -> w566
              tunnel: [w576 w593] -> w567
              tunnel: w560 -> [w575 _]
              tunnel: w565 -> [w569 _]
              tunnel: [State_Type_Definitions."Idle" ("Enum") State_Type_Definitions."Shutdown" ("Enum")] -> w559
              tunnel: w554 -> [w568 _]
              frame "None", Default {
                # ">> Manual override forces program to true stop >>"
                # ">>If ENABLE or Trigger is set to true>>"
                n223 = Or(x=w568, y=w569) -> (x .or. y?=w574:bool)
                n224 = case shown="False" w568 {
                  tunnel: [w581 w586] -> w576
                  tunnel: w575 -> [w580 w585]
                  frame False {
                    n225 = for {
                      shift-right: [w583] -> w581
                      shift-left: w580 -> [w584]
                      tunnel: string[] ["FORWARD", "READ ULTRASONIC", "READ YAW"] ("element") -> [w582] mode=indexing
                      n226 = Enqueue Element(queue=w584, element=w582) -> (queue out=w583:refnum<queue>)  [unwired: 2 in, 2 out]
                    }
                  }
                  frame True {
                    n227 = for {
                      shift-right: [w589] -> w586
                      shift-left: w585 -> [w590]
                      tunnel: string[] ["STOP", "RESET YAW", "RESET ENCODERS", "RESET FLAGS"] -> [w588] mode=indexing
                      n228 = Enqueue Element(queue=w590, element=w588) -> (queue out=w589:refnum<queue>)  [unwired: 2 in, 2 out]
                    }
                  }
                }
                n229 = Select(t=State_Type_Definitions."True Stop" ("Enum"), s=w569, f=State_Type_Definitions."Task 4_C" ("Enum")) -> (s? t:f=w571:T6)
                n230 = Select(t=w571, s=w574, f=State_Type_Definitions."Task 4_B" ("Enum")) -> (s? t:f=w578:T6)
              }
              frame "Exit" {
                n231 = for {
                  shift-right: [w596] -> w593
                  shift-left: _ -> [w597]
                  tunnel: string[] ["STOP", "RESET ENCODERS", "RESET YAW", ""] -> [w595] mode=indexing
                  n232 = Enqueue Element(queue=w597, element=w595) -> (queue out=w596:refnum<queue>)  [unwired: 2 in, 2 out]
                }
              }
            }
          }
          frame 14 {
            w607 = u8 20
            # ">> xDistance travelled>>"
            # ">> Path NOT blocked >>"
            # ">>> yStepper command>>>"
            # ">> Manual override >>"
            n233 = Dequeue Element(queue=w617, timeout in ms (-1)=w610, error in (no error)=w609) -> (element=w611:T7)  [unwired: 3 out]
            n234 = Greater?(x=w599, y=w607) -> (0:w605:bool)
            n235 = Greater?(x=w604, y=150.0) -> (0:w602:bool)
            n236 = Greater?(x=w598, y=w607) -> (0:w606:bool)
            n237 = And(x=w606, y=w605) -> (x .and. y?=w601:bool)
            n238 = And(x=w602, y=w601) -> (x .and. y?=w600:bool)
            n239 = case shown="\"None\", Default" w611 {
              tunnel: [w628 State_Type_Definitions."True Stop" ("Enum")] -> w614
              tunnel: [w626 w644] -> w613
              tunnel: w616 -> [w625 w641]
              tunnel: w615 -> [w619 _]
              tunnel: [State_Type_Definitions."Idle" ("t") State_Type_Definitions."Shutdown" ("Enum")] -> w612
              tunnel: w600 -> [w618 _]
              frame "None", Default {
                # ">> Manual override forces program to true stop >>"
                # ">>If ENABLE or Trigger is set to true>>"
                n240 = Or(x=w618, y=w619) -> (x .or. y?=w624:bool)
                n241 = case shown="True" w618 {
                  tunnel: [w631 w636] -> w626
                  tunnel: w625 -> [w629 w635]
                  frame False {
                    n242 = for {
                      shift-right: [w633] -> w631
                      shift-left: w629 -> [w634]
                      tunnel: string[] ["RIGHT", "READ YAW", "READ ENCODERS", "READ ULTRASONIC"] ("element") -> [w632] mode=indexing
                      n243 = Enqueue Element(queue=w634, element=w632) -> (queue out=w633:refnum<queue>)  [unwired: 2 in, 2 out]
                    }
                  }
                  frame True {
                    n244 = for {
                      shift-right: [w639] -> w636
                      shift-left: w635 -> [w640]
                      tunnel: string[] ["STOP", "RESET YAW", "RESET ENCODERS", "ARDUINO - ULTRASONIC"] -> [w638] mode=indexing
                      n245 = Enqueue Element(queue=w640, element=w638) -> (queue out=w639:refnum<queue>)  [unwired: 2 in, 2 out]
                    }
                  }
                }
                n246 = Select(t=State_Type_Definitions."True Stop" ("Enum"), s=w619, f=State_Type_Definitions."Task 4_D" ("Enum")) -> (s? t:f=w620:T6)
                n247 = Select(t=w620, s=w624, f=State_Type_Definitions."Task 4_C" ("Enum")) -> (s? t:f=w628:T6)
              }
              frame "Exit" {
                n248 = for {
                  shift-right: [w647] -> w644
                  shift-left: w641 -> [w648]
                  tunnel: string[] ["STOP", "RESET ENCODERS", "RESET YAW", ""] -> [w646] mode=indexing
                  n249 = Enqueue Element(queue=w648, element=w646) -> (queue out=w647:refnum<queue>)  [unwired: 2 in, 2 out]
                }
              }
            }
          }
          frame 15 {
            w667 = u8 20
            # ">> yDistance travelled>>"
            # ">> Path blocked >>"
            # ">>> yStepper command>>>"
            # ">> Manual override >>"
            n250 = Dequeue Element(queue=w658, timeout in ms (-1)=w657, error in (no error)=w656) -> (element=w668:T7)  [unwired: 3 out]
            n251 = Less?(x=w651, y=w667) -> (x < y?=w665:bool)
            n252 = Greater?(x=w655, y=200.0) -> (0:w663:bool)
            n253 = Less?(x=w650, y=w667) -> (x < y?=w666:bool)
            n254 = And(x=w666, y=w665) -> (x .and. y?=w662:bool)
            n255 = Or(x=w663, y=w662) -> (x .or. y?=w661:bool)
            n256 = case shown="\"None\", Default" w668 {
              tunnel: [w679 State_Type_Definitions."True Stop" ("Enum")] -> w654
              tunnel: [w677 w695] -> w652
              tunnel: w659 -> [w676 w692]
              tunnel: w660 -> [w670 _]
              tunnel: [State_Type_Definitions."Idle" ("t") State_Type_Definitions."Shutdown" ("Enum")] -> w653
              tunnel: w661 -> [w669 _]
              frame "None", Default {
                # ">> Manual override forces program to true stop >>"
                # ">>If ENABLE or Trigger is set to true>>"
                n257 = Or(x=w669, y=w670) -> (x .or. y?=w675:bool)
                n258 = case shown="False" w669 {
                  tunnel: [w682 w687] -> w677
                  tunnel: w676 -> [w680 w686]
                  frame False {
                    n259 = for {
                      shift-right: [w684] -> w682
                      shift-left: w680 -> [w685]
                      tunnel: string[] ["FORWARD", "READ YAW", "READ ENCODERS", "READ ULTRASONIC"] ("element") -> [w683] mode=indexing
                      n260 = Enqueue Element(queue=w685, element=w683) -> (queue out=w684:refnum<queue>)  [unwired: 2 in, 2 out]
                    }
                  }
                  frame True {
                    n261 = for {
                      shift-right: [w690] -> w687
                      shift-left: w686 -> [w691]
                      tunnel: string[] ["STOP", "RESET YAW", "RESET ENCODERS", "RESET FLAGS"] -> [w689] mode=indexing
                      n262 = Enqueue Element(queue=w691, element=w689) -> (queue out=w690:refnum<queue>)  [unwired: 2 in, 2 out]
                    }
                  }
                }
                n263 = Select(t=State_Type_Definitions."True Stop" ("Enum"), s=w670, f=State_Type_Definitions."True Stop" ("Enum")) -> (s? t:f=w671:T6)
                n264 = Select(t=w671, s=w675, f=State_Type_Definitions."Task 4_D" ("Enum")) -> (s? t:f=w679:T6)
              }
              frame "Exit" {
                n265 = for {
                  shift-right: [w698] -> w695
                  shift-left: w692 -> [w699]
                  tunnel: string[] ["STOP", "RESET ENCODERS", "RESET YAW", ""] -> [w697] mode=indexing
                  n266 = Enqueue Element(queue=w699, element=w697) -> (queue out=w698:refnum<queue>)  [unwired: 2 in, 2 out]
                }
              }
            }
          }
          frame 13 {
            # ">>> yStepper command>>>"
            # ">> Manual override >>"
            n267 = Dequeue Element(queue=w708, timeout in ms (-1)=w707, error in (no error)=w709) -> (element=w706:T7)  [unwired: 3 out]
            n268 = Equal?(x=w705, y=u8 80) -> (x = y?=w703:bool)
            n269 = case shown="\"None\", Default" w706 {
              tunnel: [w719 State_Type_Definitions."True Stop" ("Enum")] -> w710
              tunnel: [w722 w739] -> w711
              tunnel: [State_Type_Definitions."Idle" ("Enum") State_Type_Definitions."Shutdown" ("Enum")] -> w712
              tunnel: w703 -> [w718 _]
              tunnel: w702 -> [w717 _]
              tunnel: w701 -> [w713 w736]
              frame "None", Default {
                # "Stays in Task 5_A until stepper reaches desired \nheight"
                # "T: Go back to idle, F: Continue with task\""
                # ">> Manual override >>"
                n270 = case shown="True" w718 {
                  tunnel: [w726 w732] -> w722
                  tunnel: w713 -> [w724 w730]
                  frame False {
                    n271 = for {
                      tunnel: string[] ["Z STEPPER CAM HEIGHT", "READ STEPPER VALUES"] ("element") -> [w727] mode=indexing
                      shift-right: [w729] -> w726
                      shift-left: w724 -> [w728]
                      n272 = Enqueue Element(queue=w728, element=w727) -> (queue out=w729:refnum<queue>)  [unwired: 2 in, 2 out]
                    }
                  }
                  frame True {
                    n273 = for {
                      shift-right: [w734] -> w732
                      shift-left: w730 -> [w735]
                      tunnel: string[] ["ARDUINO - ULTRASONIC", "READ ULTRASONIC", ""] -> [w733] mode=indexing
                      n274 = Enqueue Element(queue=w735, element=w733) -> (queue out=w734:refnum<queue>)  [unwired: 2 in, 2 out]
                    }
                  }
                }
                n275 = Or(x=w718, y=w717) -> (x .or. y?=w720:bool)
                n276 = Select(t=State_Type_Definitions."True Stop" ("Enum"), s=w717, f=State_Type_Definitions."Task 5 _B" ("Enum")) -> (s? t:f=w714:u16)
                n277 = Select(t=w714, s=w720, f=State_Type_Definitions."Task 5_A" ("Enum")) -> (s? t:f=w719:u16)
              }
              frame "Exit" {
                n278 = for {
                  shift-right: [w742] -> w739
                  shift-left: w736 -> [w743]
                  tunnel: string[] ["STOP", "RESET ENCODERS", "RESET YAW", "ARDUINO MODE 0"] -> [w741] mode=indexing
                  n279 = Enqueue Element(queue=w743, element=w741) -> (queue out=w742:refnum<queue>)  [unwired: 2 in, 2 out]
                }
              }
            }
          }
          frame 14 {
            w749 = u8 25 ("y")
            # ">>> yStepper command>>>"
            n280 = Less?(x=w746, y=w749) -> (x < y?=w747:bool)
            n281 = Dequeue Element(queue=w753, timeout in ms (-1)=w752, error in (no error)=w754) -> (element=w751:T7)  [unwired: 3 out]
            n282 = Less?(x=w745, y=w749) -> (x < y?=w748:bool)
            n283 = And(x=w748, y=w747) -> (x .and. y?=w744:bool)
            n284 = case shown="\"None\", Default" w751 {
              tunnel: [w766 State_Type_Definitions."True Stop" ("Enum")] -> w756
              tunnel: [w769 w786] -> w755
              tunnel: [State_Type_Definitions."Idle" ("Enum") State_Type_Definitions."Shutdown" ("Enum")] -> w757
              tunnel: w759 -> [w765 _]
              tunnel: w758 -> [w761 w783]
              tunnel: w744 -> [w760 _]
              frame "None", Default {
                # "Stays in Task 5_B to capture image over 5 seconds"
                # "T: Go back to idle, F: Continue with task\""
                # ">> Manual override >>"
                n285 = case shown="True" w760 {
                  tunnel: [w773 w779] -> w769
                  tunnel: w761 -> [w771 w777]
                  frame False {
                    n286 = for {
                      tunnel: string[] ["FORWARD", "READ ULTRASONIC", "READ YAW"] ("element") -> [w774] mode=indexing
                      shift-right: [w776] -> w773
                      shift-left: w771 -> [w775]
                      n287 = Enqueue Element(queue=w775, element=w774) -> (queue out=w776:refnum<queue>)  [unwired: 2 in, 2 out]
                    }
                  }
                  frame True {
                    n288 = for {
                      shift-right: [w781] -> w779
                      shift-left: w777 -> [w782]
                      tunnel: string[] ["STOP", "RESET ENCODERS", "OPEN LOG CAM", "SET TIMER"] -> [w780] mode=indexing
                      n289 = Enqueue Element(queue=w782, element=w780) -> (queue out=w781:refnum<queue>)  [unwired: 2 in, 2 out]
                    }
                  }
                }
                n290 = Or(x=w760, y=w765) -> (x .or. y?=w767:bool)
                n291 = Select(t=State_Type_Definitions."True Stop" ("Enum"), s=w765, f=State_Type_Definitions."Task 5_C" ("Enum")) -> (s? t:f=w762:u16)
                n292 = Select(t=w762, s=w767, f=State_Type_Definitions."Task 5 _B" ("Enum")) -> (s? t:f=w766:u16)
              }
              frame "Exit" {
                n293 = for {
                  shift-right: [w789] -> w786
                  shift-left: w783 -> [w790]
                  tunnel: string[] ["STOP", "RESET ENCODERS", "RESET YAW", "ARDUINO MODE 0"] -> [w788] mode=indexing
                  n294 = Enqueue Element(queue=w790, element=w788) -> (queue out=w789:refnum<queue>)  [unwired: 2 in, 2 out]
                }
              }
            }
          }
          frame 15 {
            # ">>> yStepper command>>>"
            # ">> Manual override >>"
            n295 = Dequeue Element(queue=w799, timeout in ms (-1)=w798, error in (no error)=w797) -> (element=w796:T7)  [unwired: 3 out]
            n296 = case shown="\"None\", Default" w796 {
              tunnel: [w806 State_Type_Definitions."True Stop" ("Enum")] -> w801
              tunnel: [w809 w826] -> w794
              tunnel: [State_Type_Definitions."Idle" ("Enum") State_Type_Definitions."Shutdown" ("Enum")] -> w793
              tunnel: w795 -> [w803 _]
              tunnel: w800 -> [w805 w823]
              tunnel: w791 -> [w802 _]
              frame "None", Default {
                # ">> Is time up? >>"
                # "Determines if object is in range to pick up"
                # ">> Manual override >>"
                n297 = case shown="True" w802 {
                  tunnel: [w813 w819] -> w809
                  tunnel: w805 -> [w811 w817]
                  frame False {
                    n298 = for {
                      tunnel: string[] ["CAM ACQ", "START TIMER"] ("element") -> [w814] mode=indexing
                      shift-right: [w816] -> w813
                      shift-left: w811 -> [w815]
                      n299 = Enqueue Element(queue=w815, element=w814) -> (queue out=w816:refnum<queue>)  [unwired: 2 in, 2 out]
                    }
                  }
                  frame True {
                    n300 = for {
                      shift-right: [w821] -> w819
                      shift-left: w817 -> [w822]
                      tunnel: string[] ["CAM CLOSE", "PROCESS IMAGE"] -> [w820] mode=indexing
                      n301 = Enqueue Element(queue=w822, element=w820) -> (queue out=w821:refnum<queue>)  [unwired: 2 in, 2 out]
                    }
                  }
                }
                n302 = Or(x=w802, y=w803) -> (x .or. y?=w807:bool)
                n303 = Select(t=State_Type_Definitions."Task 5_D" ("Enum"), s=w807, f=State_Type_Definitions."Task 5_D" ("Enum")) -> (s? t:f=w806:T24)
              }
              frame "Exit" {
                n304 = for {
                  shift-right: [w829] -> w826
                  shift-left: w823 -> [w830]
                  tunnel: string[] ["STOP", "RESET ENCODERS", "RESET YAW", "ARDUINO MODE 0"] -> [w828] mode=indexing
                  n305 = Enqueue Element(queue=w830, element=w828) -> (queue out=w829:refnum<queue>)  [unwired: 2 in, 2 out]
                }
              }
            }
          }
          frame 16 {
            # ">>> yStepper command>>>"
            n306 = Dequeue Element(queue=w836, timeout in ms (-1)=w835, error in (no error)=w834) -> (element=w833:T7)  [unwired: 3 out]
            n307 = case shown="\"None\", Default" w833 {
              tunnel: [w848 State_Type_Definitions."True Stop" ("Enum")] -> w840
              tunnel: [w851 w868] -> w839
              tunnel: [State_Type_Definitions."Idle" ("Enum") State_Type_Definitions."Shutdown" ("Enum")] -> w841
              tunnel: w837 -> [w847 _]
              tunnel: w838 -> [w843 w865]
              tunnel: w831 -> [w842 _]
              frame "None", Default {
                # ">> T: Breaks out of state loop; F: Stays in loop>>"
                # ">> Manual override >>"
                # ">> Checks if object is detected>>"
                # "Stays in Task 5D until the object is detected"
                # "T: Go back to idle, F: Continue with task\""
                # ">> Manual override >>"
                n308 = case shown="True" w842 {
                  tunnel: [w855 w861] -> w851
                  tunnel: w843 -> [w853 w859]
                  frame False {
                    n309 = for {
                      tunnel: string[] ["PROCESS IMAGE", "", ""] ("element") -> [w856] mode=indexing
                      shift-right: [w858] -> w855
                      shift-left: w853 -> [w857]
                      n310 = Enqueue Element(queue=w857, element=w856) -> (queue out=w858:refnum<queue>)  [unwired: 2 in, 2 out]
                    }
                  }
                  frame True {
                    n311 = for {
                      shift-right: [w863] -> w861
                      shift-left: w859 -> [w864]
                      tunnel: string[] ["DISPOSE BUFFERS", "CAM CLOSE", ""] -> [w862] mode=indexing
                      n312 = Enqueue Element(queue=w864, element=w862) -> (queue out=w863:refnum<queue>)  [unwired: 2 in, 2 out]
                    }
                  }
                }
                n313 = Or(x=w842, y=w847) -> (x .or. y?=w849:bool)
                n314 = Select(t=State_Type_Definitions."True Stop" ("Enum"), s=w847, f=State_Type_Definitions."True Stop" ("Enum")) -> (s? t:f=w844:T6)
                n315 = Select(t=w844, s=w849, f=State_Type_Definitions."Task 5_D" ("Enum")) -> (s? t:f=w848:u16)
              }
              frame "Exit" {
                n316 = for {
                  shift-right: [w871] -> w868
                  shift-left: w865 -> [w872]
                  tunnel: string[] ["STOP", "RESET ENCODERS", "RESET YAW", "ARDUINO MODE 0"] -> [w870] mode=indexing
                  n317 = Enqueue Element(queue=w872, element=w870) -> (queue out=w871:refnum<queue>)  [unwired: 2 in, 2 out]
                }
              }
            }
          }
          frame 25 {
            # ">>> yStepper command>>>"
            n318 = Dequeue Element(queue=w880, timeout in ms (-1)=w879, error in (no error)=w878) -> (element=w885:T7)  [unwired: 3 out]
            n319 = Equal?(x=w876, y=u8 80) -> (x = y?=w875:bool)
            n320 = case shown="\"None\", Default" w885 {
              tunnel: [w892 State_Type_Definitions."True Stop" ("Enum")] -> w883
              tunnel: [w891 w909] -> w882
              tunnel: [State_Type_Definitions."Idle" ("Enum") State_Type_Definitions."Shutdown" ("Enum")] -> w884
              tunnel: w881 -> [w887 _]
              tunnel: w877 -> [w889 _]
              tunnel: w875 -> [w886 _]
              frame "None", Default {
                n321 = case shown="True" w886 {
                  tunnel: [w897 w903] -> w891
                  tunnel: w889 -> [w895 w901]
                  frame False {
                    n322 = for {
                      tunnel: string[] ["Z STEPPER CAM HEIGHT", "READ STEPPER VALUES"] ("element") -> [w898] mode=indexing
                      shift-right: [w900] -> w897
                      shift-left: w895 -> [w899]
                      n323 = Enqueue Element(queue=w899, element=w898) -> (queue out=w900:refnum<queue>)  [unwired: 2 in, 2 out]
                    }
                  }
                  frame True {
                    n324 = for {
                      shift-right: [w905] -> w903
                      shift-left: w901 -> [w906]
                      tunnel: string[] ["CAM ACQ", "OPEN LOG CAM"] -> [w904] mode=indexing
                      n325 = Enqueue Element(queue=w906, element=w904) -> (queue out=w905:refnum<queue>)  [unwired: 2 in, 2 out]
                    }
                  }
                }
                n326 = Or(x=w886, y=w887) -> (x .or. y?=w888:bool)
                n327 = Select(t=State_Type_Definitions."Task 6_B" ("Enum"), s=w888, f=State_Type_Definitions."Task 6_A" ("Enum")) -> (s? t:f=w892:T6)
              }
              frame "Exit" {
                n328 = for {
                  shift-right: [w912] -> w909
                  shift-left: _ -> [w913]
                  tunnel: string[] ["STOP", "RESET ENCODERS", "RESET YAW", "ARDUINO MODE 0"] -> [w911] mode=indexing
                  n329 = Enqueue Element(queue=w913, element=w911) -> (queue out=w912:refnum<queue>)  [unwired: 2 in, 2 out]
                }
              }
            }
          }
          frame 24 {
            # ">>> yStepper command>>>"
            n330 = Dequeue Element(queue=w923, timeout in ms (-1)=w921, error in (no error)=w922) -> (element=w920:T7)  [unwired: 3 out]
            n331 = case shown="\"None\", Default" w920 {
              tunnel: [w930 State_Type_Definitions."True Stop" ("Enum")] -> w916
              tunnel: [w929 w948] -> w924
              tunnel: [State_Type_Definitions."Idle" ("Enum") State_Type_Definitions."Shutdown" ("Enum")] -> w917
              tunnel: w919 -> [w925 _]
              tunnel: w918 -> [w927 _]
              tunnel: w915 -> [w926 w945]
              frame "None", Default {
                # ">> Manual override >>"
                n332 = case shown="True" w927 {
                  tunnel: [w935 w941] -> w929
                  tunnel: w926 -> [w934 w939]
                  frame False {
                    n333 = for {
                      shift-right: [w938] -> w935
                      shift-left: w934 -> [w937]
                      tunnel: string[] ["CAM ACQ", "PROCESS IMAGE", "OPEN CLAW"] -> [w936] mode=indexing
                      n334 = Enqueue Element(queue=w937, element=w936) -> (queue out=w938:refnum<queue>)  [unwired: 2 in, 2 out]
                    }
                  }
                  frame True {
                    n335 = for {
                      shift-right: [w943] -> w941
                      shift-left: w939 -> [w944]
                      tunnel: string[] ["CAM ACQ", "PROCESS IMAGE", "CLOSE CLAW"] -> [w942] mode=indexing
                      n336 = Enqueue Element(queue=w944, element=w942) -> (queue out=w943:refnum<queue>)  [unwired: 2 in, 2 out]
                    }
                  }
                }
                n337 = Select(t=State_Type_Definitions."True Stop" ("Enum"), s=w925, f=State_Type_Definitions."Task 6_B" ("Enum")) -> (s? t:f=w930:T6)
              }
              frame "Exit" {
                # ">> State after true stop >>"
                # ">> Goes to true stop >>"
                n338 = for {
                  shift-right: [w951] -> w948
                  shift-left: w945 -> [w952]
                  tunnel: string[] ["STOP", "RESET ENCODERS", "RESET YAW", ""] -> [w950] mode=indexing
                  n339 = Enqueue Element(queue=w952, element=w950) -> (queue out=w951:refnum<queue>)  [unwired: 2 in, 2 out]
                }
              }
            }
          }
        }
      }
    }
    n340 = local write "Green LED"(w196) -> ()
  }
  n341 = call <vilib>:"DIO Close.vi"("error in (no error)"=w24, "DIO Info In"=w27) -> ()  [unwired: 9 in, 1 out]
  n342 = call <vilib>:"DIO Close.vi"("error in (no error)"=w34, "DIO Info In"=w36) -> ()  [unwired: 9 in, 1 out]
  n343 = call <vilib>:"NavX Close.vi"("error in (no error)"=w5, "NavX Info In"=w4) -> ()  [unwired: 9 in, 1 out]
  n344 = call <vilib>:"DIO Close.vi"("error in (no error)"=w29, "DIO Info In"=w31) -> ()  [unwired: 9 in, 1 out]
  n345 = call <vilib>:"DIO Close.vi"("error in (no error)"=w12, "DIO Info In"=w13) -> ()  [unwired: 9 in, 1 out]
  n346 = call <vilib>:"DIO Close.vi"("error in (no error)"=w7, "DIO Info In"=w8) -> ()  [unwired: 9 in, 1 out]
  n347 = while {
    stop <- w1384 stop-if-true
    n348 = call <vilib>:"RT Get CPU Loads.vi"() -> ("CPU loads"=→"CPU loads":T5[])  [unwired: 10 in, 1 out]
    n349 = Wait (ms)(milliseconds to wait=u32 100) -> ()  [unwired: 1 out]
    n350 = call "FGV Bool.vi"("Init/Read/Write State"=States_for_Action_Engine."Read") -> ("Output node"=w1384:bool)  [unwired: 2 in, 1 out]
  }
  n351 = Merge Errors "Merge Errors"(w64, w63) -> (w46:errorcluster)
  n352 = Merge Errors(w50, w46) -> (w45:errorcluster)
  n353 = Destroy User Event(user event=w67, error in=w45) -> ()  [unwired: 1 out]
  n354 = Destroy User Event(user event=w68, error in=w45) -> ()  [unwired: 1 out]
  n355 = Unregister For Events(event registration refnum=w59, error in=w45) -> ()  [unwired: 1 out]
  n356 = Release Queue(queue=w41, error in (no error)=w45) -> (error out=w23:errorcluster)  [unwired: 1 in, 2 out]
  n357 = Release Queue(queue=w58, error in (no error)=w45) -> ()  [unwired: 1 in, 3 out]
  n358 = call <vilib>:"Simple Error Handler.vi"("error in (no error)"=w23) -> ("error out"=w22:errorcluster)  [unwired: 4 in, 4 out]
  n359 = call <vilib>:"Reset myRIO.vi"("error in (no error)"=w22) -> ("error out"=→"error out":errorcluster)  [unwired: 10 in]
